vi "UHR-Fleezers Control (fpga) - 11.3h-c.vi"() -> ()   [LabVIEW 2012]
doc: "UHR-Fleezers Instrument Control Code (fpga)"
uses:
  <vilib>/Platform/TimedLoop/XDataNode/timing_clust.ctl
  <vilib>/Platform/TimedLoop/XDataNode/nitl_modes.ctl
  <vilib>/Platform/TimedLoop/XDataNode/wakeup.ctl
  <vilib>/rvi/eio/common/nirviEmuTemplateMethod_errors.vi
  <vilib>/rvi/interface/RandomDataEmulation/nirviRandomDataFPGAFIFO.vi
  <vilib>/rvi/interface/RandomDataEmulation/niFpgaRandomDataHandleErrors.vi
  <vilib>/rvi/Emulation/niFpgaSctlEmulationGetInTimedLoop.vi
  <vilib>/rvi/Emulation/niFpgaSctlEmulationGlobalWrite.vi
  <vilib>/rvi/Emulation/niFpgaSctlEmulationRegisterWithScheduler.vi
  <vilib>/rvi/Emulation/niFpgaSctlEmulationScheduler.vi
  <vilib>/Platform/TimedLoop/XDataNode/XDataNode.xnode
  <vilib>/eio/EIOMethodNode/EIOMethodNode.xnode
  <vilib>/eio/EIONode/EIONode.xnode
  <vilib>/rvi/DataTransferAndStorage/Container/XNode/niFpgaContainer.xnode
  <vilib>/rvi/interface/RandomDataEmulation/nirviRandomDataFpgaReadWriteTemplate.vi
  <vilib>/addons/control/pid/fpga.llb/XNode/niFpgaPID.xnode
  <vilib>/Platform/TimedLoop/XDataNode/XDNodeRunTimeDep.lvlib
panel:
  in  "Tab Control":T1(tab)=enum."Force FB"
  in  "Set 3":bool
  in  "Set 2":bool=TRUE
  in  "Set 1":bool=TRUE
  in  "Trap Pos to FIFO":bool
  in  "N of AI1 Int Acq Sets":i16=2 min=1 max=3 step=1
  out "AI Late Counter":u8
  in  "ai count":u16=400
  in  "+ phase":bool
  in  "Phase count adjustment":i16
  out "Relative phase":i16
  in  "AI to FIFO":bool
  out "BD1 Frequency Out 1":u64
  out "BD1 Frequency Out 2":u64
  out "Trap Pos FIFO Timeout":u16
  out "Trap AI FIFO Timeout":u16
  in  "Trap FIFO Set Timeout":i32
  in  "Tab Control 2":T2(tab)
  in  "RD":bool
  in  "FB1 output high":i16=3000
  in  "FB1 output low":i16
  in  "D1":i16
  in  "I1":i16=5
  in  "P1":i16=10
  in  "Swap F1 and F2":bool
  in  "Cont. Scan":bool
  in  "Abort scan":bool
  in  "Cycles per step":u64
  in  "Scan BD":bool
  in  "Number of scans":u16
  in  "Scan steps":u64
  in  "Scan freq.  increment":i64
  out "Scanning":bool
  in  "Start scan":bool
  in  "OSK Bd 1":bool
  in  "Reset Bd 1":bool
  in  "PMODE":bool
  in  "Direct RF Box \nCommunication":bool
  in  "Data BD 2":u8 format="%08b"
  in  "Data BD 1":u8 format="%08b"
  in  "Address":u8 format="%02x"
  in  "Update Data":bool
  in  "FPGA Controls\n RF Box":bool
  in  "Number Interlace Cycles":u8=2 min=1 max=3
  in  "Interlace Off Parameters":u8=1 min=1 max=3
  in  "Interlace ON/OFF":bool
  out "DIO Relative phase":i16
  in  "Phase count adjustment (DIO)":i16
  in  "+ phase (DIO)":bool
  out "DIO Late Counter":u8
  in  "DIO count 1 (ticks)":u16=400
  in  "DIO count 2 (ticks)":u16=400
  in  "DIO count 3 (ticks)":u16=400
  out "AI2 Y Sum Set 2":i16
  out "AI2 Y Sum Set 1":i16
  in  "FB Setpoint Set 1":i16 min=0 step=1
  in  "FB Reset Set 1":bool
  in  "FB On/Off Set 1":bool
  in  "FB Reset Set 2":bool
  in  "FB On/Off Set 2":bool
  in  "FB Setpoint Set 2":i16 min=0 step=1
  out "Scan I":u64
  in  "Amp switch delay":u16=5
  in  "BD 2 Amplitude 1":u16
  in  "BD 1 Amplitude 1":u16
  in  "BD 2 Frequency 1":u64
  in  "BD 1 Frequency 1":u64
  in  "BD 2 Amplitude 2":u16
  in  "BD 1 Amplitude 2":u16
  in  "BD 2 Frequency 2":u64
  in  "BD 1 Frequency 2":u64
  in  "BD 2 Amplitude 3":u16
  in  "BD 1 Amplitude 3":u16
  in  "BD 2 Frequency 3":u64
  in  "BD 1 Frequency 3":u64
  in  "FB2 output high":fxp<+/-,16,1>=0.999969482421875
  in  "FB2 output low":fxp<+/-,16,1>=-1.0
  in  "P2":fxp<+/-,16,8> format="%.11g"
  in  "I2":fxp<+/-,16,8>=10.0 format="%.11g"
  in  "D2":fxp<+/-,16,8> format="%.11g"
  in  "Negate Diff?":bool
  in  "Diff FB Measurement?":bool
  in  "FB Trig Integrate":u32=1
  out "TTrig?":bool
  in  "TTrig Negate Pos":bool=TRUE
  out "Trap Pos FB Int Signal":fxp<+/-,24,9> format="%.18g"
  out "Trap Pos FB Int-Norm Signal":fxp<+/-,16,1> format="%.16g"
  in  "FPGA TTrig Thresh":i64
  in  "FPGA Trap Trig":bool
  out "Trap Pos FB Action":i64
  in  "Trap Pos. FB Offset Factor":i64
  in  "Trap Pos. FB Mult Factor":i64=2
  in  "Trap Pos. FB Reset":bool
  in  "Trap Pos FB Monitor T1 or T2":bool
  in  "AI1 X Scale":u16
  in  "Trap Pos FB Int Count":u16=100
  in  "Trap Pos FB Negate Action":bool
  out "AI1 X Set 2":fxp<+/-,16,1>
  out "AI1 X Set 1":fxp<+/-,16,1>
  in  "Trap Pos. FB SP":fxp<+/-,16,1>
  in  "Force feedback":bool
  out "TTrig Sig":i64
  out "TTrig Fin Thresh":i64
  in  "1D or 2D Scan?":bool
  in  "Abort scan (MCL)":bool
  in  "MCL Scan Axis":bool
  in  "Cont. Scan (MCL)":bool
  out "Scan I (MCL)":u64
  in  "Number of scans (MCL)":u16
  out "Scanning MCL":bool
  in  "Scan steps (MCL)":u64
  in  "Cycles per step (MCL)":u64
  in  "Scan freq.  increment (MCL)":i16
  in  "Start scan (MCL)":bool
  in  "AO2":i16
  in  "AO1":i16
  out "MCL Late Counter":u8
  in  "MCL count":u32=800
  out "MCL Relative Phase":i16
  in  "Phase count adjustment (MCL)":i16
  in  "+ phase (MCL)":bool
  out "APD3 out state":bool
  in  "APD Gate Operating Mode":u8 max=2 step=1
  in  "Invert APD Gate":bool
  in  "APD Gate OFF Count":u16=100
  in  "APD Gate ON Count":u16=300
  out "APD 1 Gate Late Counter":u8
  out "APD 1 Gate Relative Phase":i16
  in  "Phase count adjustment (APD 1 Gate)":i16
  in  "+ phase (APD 1 Gate)":bool
  out "APD 2 Counts 0":u32
  out "APD 2 Counts 1":u32
  out "APD 1 Counts 0":u32
  out "APD 1 Counts 1":u32
  out "APD1 out state":bool
  in  "APD AO scale factor":i16=1
  in  "APD to FIFO":bool
  in  "APD Acq Rate Count":u32=20000000
  out "APD Acq Late Counter":u8
  out "APD Acq Relative Phase":i16
  in  "Phase Count Adjustment (APD Acq)":i16
  in  "+ phase (APD Acq)":bool
  in  "Phase count adjustment (APD 2 Gate)":i16
  out "APD 2 Gate Late Counter":u8
  out "APD 2 Gate Relative Phase":i16
  in  "+ phase (APD 2 Gate)":bool
  out "APD2 out state":bool
  out "APD 3 Counts 0":u32
  out "APD 3 Counts 1":u32
  out "APD 3 Gate Late Counter":u8
  in  "Phase count adjustment (APD 3 Gate)":i16
  out "APD 3 Gate Relative Phase":i16
  in  "+ phase (APD 3 Gate)":bool
  in  "D3":i16
  in  "I3":i16=5
  in  "P3":i16=10
  in  "Green Filter Flipper":bool
  in  "Green FB Count":u16=1200
  out "Green Late Counter":u8
  out "Green FB Relative Phase":i16
  in  "Phase count adjustment (Green FB)":i16=10
  in  "+ phase (Green FB)":bool
  out "Green FB Sum":i16
  in  "Green int current ON count adj":u16=150
  in  "Current Out":u16=30000
  in  "Green FB On/Off":bool
  in  "Green FB Setpoint":i16=250 min=0 step=1
  in  "Green FB Reset":bool
  in  "Operating Mode 2":u8=2 max=2 step=1
  in  "Invert GI 2":bool
  in  "Green interlace OFF count 2":u16=900
  in  "Green interlace ON count 2":u16=300
  out "GI Late Counter 2":u8
  out "GI Relative phase 2":i16
  in  "Phase count adjustment (GI) 2":i16=20
  in  "+ phase (GI) 2":bool
  in  "Green interlace OFF count":u16=100
  out "GI Relative phase":i16
  in  "Phase count adjustment (GI)":i16
  in  "+ phase (GI)":bool
  in  "Green interlace ON count":u16=300
  out "GI Late Counter":u8
  in  "Invert GI":bool
  in  "Operating Mode":u8 max=2 step=1
  in  "+ phase (RI)":bool
  out "RI Relative phase":i16
  out "RI Late Counter":u8
  in  "Red interlace ON count":u16=300
  in  "Red interlace OFF count":u16=100
  in  "Invert RI":bool
  in  "Red Laser Operating Mode":u8 max=2 step=1
  in  "Phase count adjustment (RI)":i16
  out "Red FB Intensity":i16
  in  "Phase count adjustment (Red FB)":i16=10
  in  "Red FB Count":u16=1200
  out "Red Late Counter":u8
  out "Red FB Relative Phase":i16
  in  "+ phase (Red FB)":bool
  in  "Phase count adjustment (RI) 2":i16=20
  in  "Red int current ON count adj":u16=150
  in  "RI Current Out":u16=30000
  in  "Red FB On/Off":bool
  in  "D4":i16
  in  "I4":i16=5
  in  "P4":i16=10
  in  "Red FB Setpoint":i16=250 min=0 step=1
  in  "Red FB Reset":bool
  in  "RI Operating Mode 2":u8=2 max=2 step=1
  in  "Invert RI 2":bool
  in  "Red interlace OFF count 2":u16=900
  in  "Red interlace ON count 2":u16=300
  out "RI Late Counter 2":u8
  out "RI Relative phase 2":i16
  in  "+ phase (RI) 2":bool
  in  "Phase count adjustment (BI AO)":i16=20
  in  "Blue current ON count adj (AO)":u16=150
  in  "BI Current Out":i16=30000
  in  "Blue FB On/Off":bool
  in  "D5":i16
  in  "I5":i16=5
  in  "P5":i16=10
  in  "Blue FB Setpoint":i16=250 min=0 step=1
  in  "Blue FB Reset":bool
  in  "BI Operating Mode (AO)":u8=2 max=2 step=1
  in  "Invert BI (AO)":bool
  in  "Blue OFF count (AO)":u16=900
  in  "Blue ON count (AO)":u16=300
  out "BI Late Counter (AO)":u8
  out "BI Relative phase (AO)":i16
  in  "+ phase (BI AO)":bool
  in  "Phase count adjustment (BI D)":i16
  in  "Blue Laser Operating Mode (D)":u8 max=2 step=1
  in  "Invert BI (D)":bool
  in  "Blue interlace OFF count (D)":u16=100
  in  "Blue interlace ON count (D)":u16=300
  out "Blue Late Counter (D)":u8
  out "BI Relative phase (D)":i16
  in  "+ phase (BI D)":bool
  out "Blue Intensity":i16
  in  "Phase count adjustment (Blue Int)":i16=10
  in  "Blue Int Count":u16=1200
  out "Blue Int Late Counter":u8
  out "Blue Int Relative Phase":i16
  in  "+ phase (Blue Int)":bool
  # "Only one of these can be on\nat a time:"
  # "Raster Scan AOD"
  # "1 (X)"
  # "2 (Y)"
  # "IR Intensity Feedback (RF BD 1)"
  # "FB Gains Set 1"
  # "FB output range 1"
  # "FB Triggering Excitation Laser"
  # "Trap Pos. FB Gains"
  # "Trap Pos. FB Range"
  # "AO1 (Y)"
  # "2D"
  # "1D"
  # "AO2 (X)"
  # "APD AO for aligning"
  # "Detection Loop"
  # "Green fluorescent laser digital gate interlacing loop"
  # "0 Forced ON\n1 Forced OFF\n2 Interlacing"
  # "Green FB Gains"
  # "Red fluorescent laser digital gate interlacing loop"
  # "Detection Loop"
  # "0 Forced ON\n1 Forced OFF\n2 Interlacing"
  # "Analog/FB Control Loop\n(Disabled)"
  # "Digital Control Loop"
  # "Blue laser intensity reading"
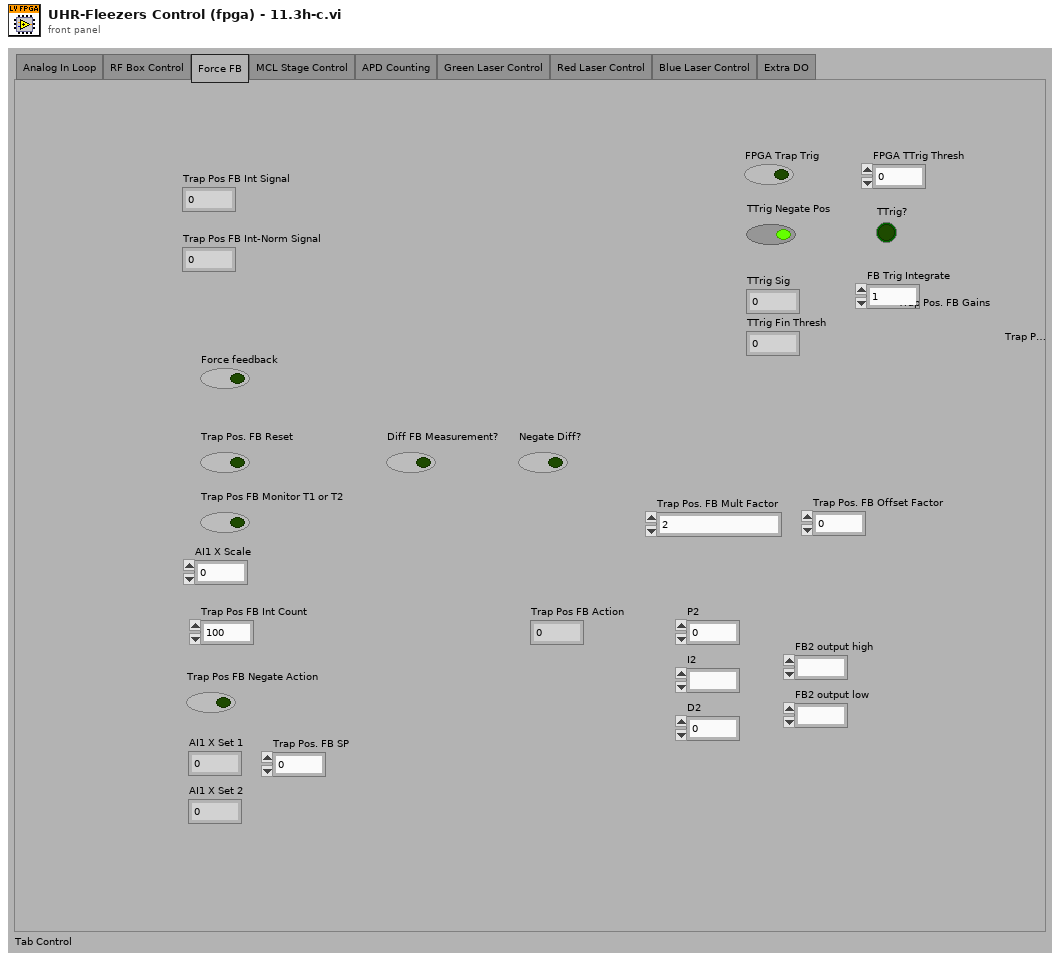
[diagram p1: front panel]
types:
  T1 = enum32{"Analog In Loop", "RF Box Control", "Force FB", "MCL Stage Control", "APD Counting", "Green Laser Control", "Red Laser Control", "Blue Laser Control", "Extra DO"}
  T2 = enum32{"Controls", "Interlacing Frequency and Amplitude Values"}
  T3 = typedef "XDNodeRunTimeDep.lvlib/timing_clust.ctl" = cluster{"Expected End [f-1]":u64, "Actual End [f-1]":u64, "Finished Late? [f-1]":bool, "Expected End [i-1]":u64, "Actual End [i-1]":u64, "Finished Late? [i-1]":bool, "Expected Start [i]":u64, "Actual Start [i]":u64, "Expected Start [f]":u64, "Actual Start [f]":u64, "Source Name":string, "Structure Name":string, "Period":i64, "Deadline":i64, "Offset":i64, "Start":i64, "Priority":i32, "Timeout":i32, "Mode":T4, "Wakeup Reason":T5, "Error":errorcluster, "Source Type":string, "Secondary Source Type":string, "Global End Time":u64, "Global Start Time":u64, "Frame Duration":u64, "Iteration Duration":u64, "Assigned CPU":i32, "I/O Scan Engine Mode":u32}
  T4 = typedef "XDNodeRunTimeDep.lvlib/nitl_modes.ctl" = enum32{"No Change", "Process missed periods, maintain original phase", "Discard missed periods, maintain original phase", "Process missed periods, ignore original phase", "Discard missed periods, ignore original phase"}
  T5 = typedef "XDNodeRunTimeDep.lvlib/wakeup.ctl" = enum32{"Normal", "Aborted", "Asynchronous wakeup", "Timing source error", "Timed loop error", "Timeout"}
  T6 = cluster{"proportional gain (Kc)":i16, "integral gain (Kc*Ts/Ti)":i16, "derivative gain (Kc*Td/Ts)":i16}
  T7 = cluster{"FB1 output high":i16, "FB1 output low":i16}
  T8 = cluster{"P2":fxp<+/-,16,8>, "I2":fxp<+/-,16,8>, "D2":fxp<+/-,16,8>}
  T9 = cluster{"FB2 output high":fxp<+/-,16,1>, "FB2 output low":fxp<+/-,16,1>}
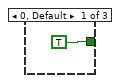
[diagram p3: hidden frame]
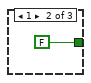
[diagram p4: hidden frame]
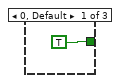
[diagram p5: hidden frame]
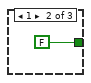
[diagram p6: hidden frame]
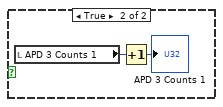
[diagram p7: hidden frame]
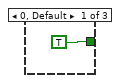
[diagram p8: hidden frame]
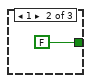
[diagram p9: hidden frame]
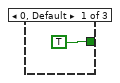
[diagram p11: hidden frame]
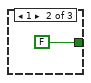
[diagram p12: hidden frame]
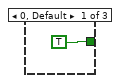
[diagram p13: hidden frame]
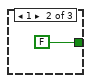
[diagram p14: hidden frame]
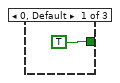
[diagram p15: hidden frame]
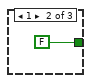
[diagram p16: hidden frame]
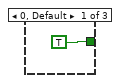
[diagram p18: hidden frame]
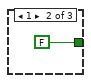
[diagram p19: hidden frame]
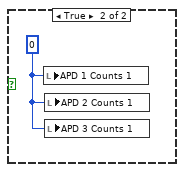
[diagram p20: hidden frame]
diagram:
  w3 = FALSE
  # "timing array current index"
  # "timing array"
  # "timing counter (phase adjusted here)"
  # "late counter"
  n1 = flat-sequence "FPGA initialization to do before running any of the loops" {
    tunnel: [u16 0 ("DIO count 3 (ticks)")] -> w2
    tunnel: [w12] -> _
    frame #0 {
      # "Start up expansion chassis early\nto avoid delays later"
      # "This pin controls udclk on the RF boards.\nWhen initially configuring the boards, this pin needs to be\nconfigured as a high impedance input.  Later it will be switched\nto an output."
      # "Initial setting of DIO data and \naddress to low (before reset).  \nThis needs to happen before the other\ncontrol method loops execute."
      n2 = xnode "FPGA I/O Node"("Chassis2/Mod4/AO0"=u16 0) -> ("Chassis2/Mod1/AI0"=w12:i16)  [unwired: 2 in, 2 out]
      n3 = xnode "FPGA I/O Method Node"("Enable"=FALSE) -> ()  [unwired: 1 in, 1 out]
      n4 = xnode "FPGA I/O Node"("Connector1/DIO0"=FALSE, "Connector1/DIO1"=FALSE, "Connector1/DIO2"=FALSE, "Connector1/DIO3"=FALSE, "Connector1/DIO4"=FALSE, "Connector1/DIO5"=FALSE, "Connector1/DIO6"=FALSE, "Connector1/DIO7"=FALSE, "Connector1/DIO8"=FALSE, "Connector1/DIO9"=FALSE, "Connector1/DIO10"=FALSE, "Connector1/DIO11"=FALSE, "Connector1/DIO12"=FALSE, "Connector1/DIO13"=FALSE, "Connector1/DIO15"=FALSE, "Connector1/DIO20"=FALSE, "Connector1/DIO21"=FALSE, "Connector1/DIO22"=FALSE, "Connector1/DIO23"=FALSE, "Connector1/DIO24"=FALSE, "Connector1/DIO25"=FALSE, "Connector1/DIO26"=FALSE, "Connector1/DIO27"=FALSE, "Connector1/DIO14"=FALSE) -> ()  [unwired: 24 in, 24 out]
    }
  }
  n5 = local read "AO1"() -> (w9:i16)
  n6 = local read "AO2"() -> (w8:i16)
  n7 = node-c288() -> (w7:T3)  [unwired: 1 in]
  n8 = timed-loop "RF box board DIO control: control bits" {
    timing: w7 -> [_]
    timing-out: [_] -> w6
    tunnel: [w42] -> _
    tunnel: w2 -> [w42]
    stop <- FALSE stop-if-true
    n9 = xnode "FPGA I/O Node"("Connector1/DIO16"="RD", "Connector1/DIO17"="PMODE", "Connector1/DIO18"="OSK Bd 1", "Connector1/DIO19"="Reset Bd 1", "Connector0/DIO3"="Green Filter Flipper") -> ()  [unwired: 5 in, 5 out]
  }
  n10 = while "RF box board DIO control: parallel communication" {
    shift-right: [w55] -> _
    shift-left: w2 -> [w54]
    shift-right: [w53] -> _
    shift-left: FALSE ("Swap F1 and F2") -> [w52]
    stop <- FALSE stop-if-true
    n11 = flat-sequence {
      tunnel: w52 -> [w59]
      tunnel: w54 -> [w57]
      tunnel: [w59] -> w51
      tunnel: [w58] -> w50
      tunnel: [w57] -> w49
      tunnel: [w65] -> w55
      tunnel: [w64] -> w53
      tunnel: w51 -> [w63]
      tunnel: w50 -> [w61]
      tunnel: w49 -> [w60]
      frame #0 {
        n12 = call "Loop Timer"("Count(Ticks)"=w57) -> ("Tick Count(Ticks)"=w58:u16)
      }
      frame #1 {
        n13 = flat-sequence {
          tunnel: ["FPGA Controls\n RF Box"] -> w62
          tunnel: w63 -> [w66]
          tunnel: [w106] -> w65
          tunnel: [w119] -> w64
          tunnel: w62 -> [w118]
          tunnel: w61 -> [w112]
          tunnel: w60 -> [w109]
          frame #0 {
            n14 = case shown="True" "FPGA Controls\n RF Box" {
              tunnel: w66 -> [_ w68]
              frame False {
              }
              frame True {
                n15 = flat-sequence {
                  tunnel: w68 -> [w74]
                  frame #0 {
                    n16 = First Call?() -> (First Call?: T/F=w69:bool)
                    n17 = case shown="True" w69 {
                      frame False {
                      }
                      frame True {
                        # "If first time data updated, be sure to set WR high and UDCLK low\nbefore setting data and address bits."
                        n18 = xnode "FPGA I/O Method Node"("Enable"=TRUE) -> ("FPGA I/O Out"=w71:refnum<k21>)  [unwired: 1 in]
                        n19 = xnode "FPGA I/O Node"("Connector1/DIO15"=TRUE) -> ()  [unwired: 1 in, 1 out]
                        n20 = xnode "FPGA I/O Node"("I/O Item"=FALSE ("Connector1/DIO30"), "FPGA I/O In"=w71) -> ()  [unwired: 1 out]
                      }
                    }
                  }
                  frame #1 {
                    n21 = flat-sequence {
                      tunnel: w74 -> [w75]
                      frame #0 {
                        # "switch frequency"
                        n22 = xnode "FPGA I/O Node"("Connector1/DIO36"=w75) -> ()  [unwired: 1 in, 1 out]
                      }
                      frame #1 {
                        n23 = call "Wait4"("Count(Ticks)"="Amp switch delay") -> ()  [unwired: 1 out]
                      }
                      frame #2 {
                        # "switch amplitude"
                        # "send udclk high"
                        n24 = xnode "FPGA I/O Node"("Connector1/DIO30"=TRUE ("Connector1/DIO15")) -> ()  [unwired: 1 in, 1 out]
                      }
                      frame #3 {
                        # "send udclk low"
                        n25 = xnode "FPGA I/O Node"("Connector1/DIO30"=FALSE ("Connector1/DIO15")) -> ()  [unwired: 1 in, 1 out]
                      }
                    }
                  }
                }
              }
            }
          }
          frame #1 {
            # "This is the prior cycle's on time"
            # "increment timing\nindex, reset to 0 if \nend of matrix"
            # "Reset to begginning (1) when number of cycles reached."
            # "timing index"
            # "build byte stacks for writing data\n(must correspond to addresses array constant)"
            # "Timing housekeeping"
            # "Adjust phase if late\n(maintains constant phase relationship between cycles)"
            n26 = Bundle("FB1 output high"="FB1 output high", "FB1 output low"="FB1 output low") -> (w79:T7)  [unwired: 1 in]
            n27 = Bundle("P1"="P1", "I1"="I1", "D1"="D1") -> (w80:cluster{"P1":i16, "I1":i16, "D1":i16})  [unwired: 1 in]
            n28 = feedback #1(u8 0 ("t")) -> (w115:u8)
            n29 = Increment(x=w115) -> (x+1=w159:u8)
            n30 = Increment(x="Number Interlace Cycles") -> (x+1=w154:u8)
            n31 = Equal?(x=w159, y=w154) -> (x = y?=w161:bool)
            n32 = Select(t=u8 1, s=w161, f=w159) -> (s? t:f=w114:u8)
            n33 = feedback-in #1(w114) -> ()
            n34 = Increment(x=w114) -> (x+1=w156:u8)
            n35 = Equal?(x=w156, y=w154) -> (x = y?=w157:bool)
            n36 = Select(t=u8 1, s=w157, f=w156) -> (s? t:f=w153:u8)
            n37 = Select(t=w153, s="Interlace ON/OFF", f="Interlace Off Parameters") -> (s? t:f=w137:u8)
            n38 = case shown="1, Default" w137 {
              tunnel: [w233 "BD 1 Frequency 2" "BD 1 Frequency 3"] -> w149
              tunnel: [w232 "BD 2 Frequency 2" "BD 2 Frequency 3"] -> w138
              tunnel: ["BD 2 Amplitude 1" "BD 2 Amplitude 2" "BD 2 Amplitude 3"] -> w94
              tunnel: [w221 w392 "BD 1 Amplitude 3"] -> w97
              tunnel: w80 -> [w195 w389 _]
              tunnel: w79 -> [w196 w388 _]
              frame 1, Default {
                w212 = fxp<+/-,24,9> 0.0 ("AI1 X Set 2")
                w205 = u16 0
                w228 = u64 0 ("f")
                # "This signal integration happens no matter what\nso that correct setpoints can be chosen before \nturning on the FB."
                # "Trap 1"
                n39 = local read "AI1 X Set 2"() -> (w208:fxp<+/-,16,1>)
                n40 = local read "AI1 X Set 1"() -> (w209:fxp<+/-,16,1>)
                n41 = local read "Scanning"() -> (w234:bool)
                n42 = Or(x=w234, y="Start scan") -> (x .or. y?=w226:bool)
                n43 = case shown="False" "Diff FB Measurement?" {
                  tunnel: w208 -> [w242 w251]
                  tunnel: w209 -> [w241 w252]
                  tunnel: [w239 w243] -> w210
                  frame False {
                    n44 = Select(t=w241, s="Trap Pos FB Monitor T1 or T2", f=w242) -> (s? t:f=w239:fxp<+/-,16,1>)
                  }
                  frame True {
                    n45 = Subtract(x=w252, y=w251) -> (x-y=w244:fxp<+/-,17,2>)
                    n46 = Not(x="Negate Diff?") -> (.not. x?=w250:bool)
                    n47 = Boolean To (0,1)(Boolean="Negate Diff?") -> (0, 1=w248:i16)
                    n48 = Boolean To (0,1)(Boolean=w250) -> (0, 1=w249:i16)
                    n49 = Negate(x=w248) -> (-x=w247:i16)
                    n50 = Add(x=w247, y=w249) -> (x+y=w245:i16)
                    n51 = Multiply(x=w245, y=w244) -> (x*y=w243:fxp<+/-,32,17>)
                  }
                }
                n52 = Not(x="Abort scan") -> (.not. x?=w224:bool)
                n53 = And(x=w224, y=w226) -> (x .and. y?=w223:bool)
                n54 = case "For raster scanning" shown="True" w223 {
                  tunnel: [u64 0 w378] -> w229
                  tunnel: "Start scan" -> [_ w363]
                  frame False {
                    n55 = local write "Scanning"(FALSE ("scanning")) -> ()
                  }
                  frame True {
                    w347 = i64 0
                    w346 = u64 0
                    # "scan incr."
                    # "freq. incr. mult."
                    # "count steps"
                    # "count number of cycles"
                    n56 = feedback #2(w346) -> (w375:u64)
                    n57 = Select(t=w346, s=w363, f=w375) -> (s? t:f=w377:u64)
                    n58 = Increment(x=w377) -> (x+1=w374:u64)
                    n59 = Greater?(x="Cycles per step", y=w374) -> (0:w356:bool)
                    n60 = Select(t=w374, s=w356, f=w346) -> (s? t:f=w373:u64)
                    n61 = feedback-in #2(w373) -> ()
                    n62 = feedback #3(w346) -> (w372:u64)
                    n63 = Select(t=w346, s=w363, f=w372) -> (s? t:f=w367:u64)
                    n64 = Increment(x=w367) -> (x+1=w371:u64)
                    n65 = Add(x="Scan steps", y="Scan steps") -> (x+y=w370:u64)
                    n66 = Select(t=w367, s=w356, f=w371) -> (s? t:f=w351:u64)
                    n67 = Greater?(x=w370, y=w351) -> (0:w350:bool)
                    n68 = Select(t=w351, s=w350, f=w346) -> (s? t:f=w368:u64)
                    n69 = feedback-in #3(w368) -> ()
                    n70 = Equal?(x="Scan steps", y=w351) -> (x = y?=w355:bool)
                    n71 = Greater?(x="Scan steps", y=w367) -> (0:w366:bool)
                    n72 = feedback #4(w347) -> (w369:i64)
                    n73 = Select(t=w347, s=w363, f=w369) -> (s? t:f=w353:i64)
                    n74 = Increment(x=w353) -> (x+1=w365:i64)
                    n75 = Decrement(x=w353) -> (x-1=w364:i64)
                    n76 = Select(t=w365, s=w366, f=w364) -> (s? t:f=w354:i64)
                    n77 = Select(t=w353, s=w355, f=w354) -> (s? t:f=w352:i64)
                    n78 = Select(t=w353, s=w356, f=w352) -> (s? t:f=w348:i64)
                    n79 = Select(t=w348, s=w350, f=w347) -> (s? t:f=w349:i64)
                    n80 = feedback-in #4(w349) -> ()
                    n81 = feedback #5(w346) -> (w362:u64)
                    n82 = Select(t=w346, s=w363, f=w362) -> (s? t:f=w358:u64)
                    n83 = Increment(x=w358) -> (x+1=w359:u64)
                    n84 = Select(t=w358, s=w350, f=w359) -> (s? t:f=w357:u64)
                    n85 = Greater?(x="Number of scans", y=w357) -> (0:w343:bool)
                    n86 = Multiply(x="Scan freq.  increment", y=w353) -> (x*y=w378:i64)
                    n87 = Select(t=TRUE, s="Cont. Scan", f=w343) -> (s? t:f=w342:bool)
                    "Scanning" <- w342
                    n88 = Select(t=w357, s=w342, f=w346) -> (s? t:f=w360:u64)
                    n89 = feedback-in #5(w360) -> ()
                    n90 = Increment(x=w357) -> (x+1=→"Scan I":u64)
                  }
                }
                n91 = feedback #6(w205) -> (w204:u16)
                n92 = Increment(x=w204) -> (x+1=w206:u16)
                n93 = Greater Or Equal?(x=w206, y="Trap Pos FB Int Count") -> (x >= y?=w197:bool)
                n94 = Select(t=w205, s=w197, f=w206) -> (s? t:f=w207:u16)
                n95 = feedback-in #6(w207) -> ()
                n96 = feedback #7(w212) -> (w211:fxp<+/-,24,9>)
                n97 = Add(x=w210, y=w211) -> (x+y=w203:fxp<+/-,24,9>)
                n98 = case "For intensity feedback" shown="True" "FB On/Off Set 1" {
                  tunnel: "BD 1 Amplitude 1" -> [w380 _]
                  tunnel: [w380 w384] -> w221
                  tunnel: w196 -> [_ w381]
                  tunnel: w195 -> [_ w382]
                  frame False {
                  }
                  frame True {
                    n99 = local read "AI2 Y Sum Set 1"() -> (w385:i16)
                    n100 = call "Slower PID.vi"("process variable"=w385, "reset?"="FB Reset Set 1", "setpoint"="FB Setpoint Set 1", "PID gains (x 2^8)"=w382, "output range"=w381) -> ("output"=w386:i16)  [unwired: 10 out]
                    n101 = To Unsigned Word Integer(number=w386) -> (unsigned 16bit integer=w384:u16)
                  }
                }
                n102 = Select(t=w212, s=w197, f=w203) -> (s? t:f=w215:fxp<+/-,24,9>)
                n103 = feedback-in #7(w215) -> ()
                n104 = Divide(x=w203, y="Trap Pos FB Int Count") -> (x/y=w198:fxp<+/-,16,1>)
                n105 = feedback #8(fxp<+/-,24,9> 0.0 ("AI1 X Set 2")) -> (w216:fxp<+/-,24,9>)
                n106 = Select(t=w203, s=w197, f=w216) -> (s? t:f=w217:fxp<+/-,24,9>)
                "Trap Pos FB Int Signal" <- w217
                n107 = feedback-in #8(w217) -> ()
                n108 = feedback #9(fxp<+/-,16,1> 0.0 ("Trap Pos FB Int-Norm Signal")) -> (w200:fxp<+/-,16,1>)
                n109 = Select(t=w198, s=w197, f=w200) -> (s? t:f=w199:fxp<+/-,16,1>)
                "Trap Pos FB Int-Norm Signal" <- w199
                n110 = feedback-in #9(w199) -> ()
                n111 = case "For position feedback" shown="True" "Force feedback" {
                  tunnel: [i64 0 w258] -> w218
                  tunnel: w198 -> [_ w255]
                  tunnel: w197 -> [_ w254]
                  frame False {
                  }
                  frame True {
                    n112 = feedback #10(i64 0) -> (w257:i64)
                    n113 = case shown="True" w254 {
                      tunnel: [w259 w273] -> w258
                      tunnel: w257 -> [w259 _]
                      tunnel: w255 -> [_ w267]
                      frame False {
                      }
                      frame True {
                        w277 = u32 0
                        n114 = Bundle("P2"="P2", "I2"="I2", "D2"="D2") -> (w263:T8)  [unwired: 1 in]
                        n115 = Bundle("FB2 output high"="FB2 output high", "FB2 output low"="FB2 output low") -> (w260:T9)  [unwired: 1 in]
                        n116 = xnode ("PID")("process variable"=w267, "reset?"="Trap Pos. FB Reset", "setpoint"="Trap Pos. FB SP", "PID gains"=w263, "output range"=w260) -> ("output"=w289:fxp<+/-,16,1>)
                        n117 = Negate(x=w289) -> (-x=w288:fxp<+/-,17,2>)
                        n118 = Select(t=w288, s="Trap Pos FB Negate Action", f=w289) -> (s? t:f=w285:fxp<+/-,17,2>)
                        n119 = Scale By Power Of 2(n=u32 15, x=u32 1) -> (x*2^n=w282:u32)
                        n120 = Multiply(x=w285, y=w282) -> (x*y=w281:fxp<+/-,17,17>)
                        n121 = To Quad Integer(1:w281) -> (0:w293:i64)
                        "Trap Pos FB Action" <- w293
                        n122 = Multiply(x=w293, y="Trap Pos. FB Mult Factor") -> (x*y=w291:i64)
                        n123 = Add(x=w291, y="Trap Pos. FB Offset Factor") -> (x+y=w273:i64)
                        n124 = feedback #11() -> (w274:i64)  [unwired: 1 in]
                        n125 = Add(x=w273, y=w274) -> (x+y=w271:i64)
                        n126 = feedback #12(w277) -> (w279:u32)
                        n127 = Increment(x=w279) -> (x+1=w268:u32)
                        n128 = Greater Or Equal?(x=w268, y="FB Trig Integrate") -> (x >= y?=w269:bool)
                        n129 = Select(t=i64 0, s=w269, f=w271) -> (s? t:f=w275:i64)
                        n130 = feedback-in #11(w275) -> ()
                        n131 = Select(t=w277, s=w269, f=w268) -> (s? t:f=w278:u32)
                        n132 = feedback-in #12(w278) -> ()
                        n133 = And(x=w269, y="FPGA Trap Trig") -> (x .and. y?=w276:bool)
                        n134 = case "Trap FB trigger excitation laser ON" shown="True" w276 {
                          tunnel: w271 -> [_ w297]
                          tunnel: w268 -> [_ w295]
                          frame False {
                          }
                          frame True {
                            n135 = Not(x="TTrig Negate Pos") -> (.not. x?=w304:bool)
                            n136 = Boolean To (0,1)(Boolean="TTrig Negate Pos") -> (0, 1=w302:i16)
                            n137 = Boolean To (0,1)(Boolean=w304) -> (0, 1=w303:i16)
                            n138 = Negate(x=w302) -> (-x=w301:i16)
                            n139 = Add(x=w301, y=w303) -> (x+y=w300:i16)
                            n140 = Multiply(x=w300, y=w297) -> (x*y=w299:i64)
                            "TTrig Sig" <- w299
                            n141 = Multiply(x="FPGA TTrig Thresh", y=w295) -> (x*y=w296:i64)
                            "TTrig Fin Thresh" <- w296
                            n142 = Greater Or Equal?(x=w299, y=w296) -> (x >= y?=w298:bool)
                            n143 = case shown="True" w298 {
                              frame False {
                              }
                              frame True {
                                w307 = TRUE ("Green FB On/Off")
                                w309 = u8 2 ("Operating Mode")
                                n144 = local write "Operating Mode 2"(w309) -> ()
                                n145 = local write "Operating Mode"(w309) -> ()
                                n146 = local write "Green FB On/Off"(w307) -> ()
                                n147 = local write "FPGA Trap Trig"(FALSE ("FPGA Trap Trig")) -> ()
                                "TTrig?" <- w307
                              }
                            }
                          }
                        }
                      }
                    }
                    n148 = feedback-in #10(w258) -> ()
                  }
                }
                n149 = Select(t=w228, s="Scan BD", f=w229) -> (s? t:f=w227:u64)
                n150 = Select(t=w229, s="Scan BD", f=w228) -> (s? t:f=w230:u64)
                n151 = Add(x=w227, y="BD 2 Frequency 1") -> (x+y=w232:u64)
                n152 = Compound Arithmetic op=ADD("BD 1 Frequency 1", w218, w230) -> (w233:u64)
                "BD1 Frequency Out 1" <- w233
              }
              frame 2 {
                # "Trap 2"
                n153 = case shown="True" "FB On/Off Set 2" {
                  tunnel: [w396 w399] -> w392
                  tunnel: "BD 1 Amplitude 2" -> [w396 _]
                  tunnel: w389 -> [_ w398]
                  tunnel: w388 -> [_ w397]
                  frame False {
                  }
                  frame True {
                    n154 = local read "AI2 Y Sum Set 2"() -> (w402:i16)
                    n155 = call "Slower PID.vi"("process variable"=w402, "reset?"="FB Reset Set 2", "setpoint"="FB Setpoint Set 2", "PID gains (x 2^8)"=w398, "output range"=w397) -> ("output"=w400:i16)  [unwired: 10 out]
                    n156 = To Unsigned Word Integer(number=w400) -> (unsigned 16bit integer=w399:u16)
                  }
                }
                "BD1 Frequency Out 2" <- "BD 1 Frequency 2"
              }
              frame 3 {
                # "Fluorescence period"
              }
            }
            n157 = feedback-in #13(w112) -> ()
            n158 = feedback #13(w112) -> (w111:u16)
            n159 = Select(t=w114, s="Interlace ON/OFF", f="Interlace Off Parameters") -> (s? t:f=w152:u8)
            n160 = Subtract(x=w112, y=w111) -> (x-y=w110:u16)
            n161 = Subtract "The error"(x=w110, y=w109) -> (x-y=w87:u16)
            n162 = case shown="1, Default" w152 {
              tunnel: ["DIO count 1 (ticks)" "DIO count 2 (ticks)" "DIO count 3 (ticks)"] -> w108
              frame 1, Default {
              }
              frame 2 {
              }
              frame 3 {
              }
            }
            n163 = Number To Boolean Array(number=w87) -> (Boolean array=w88:bool[])
            n164 = Or Array Elements(Boolean array=w88) -> (logical OR=w86:bool)
            n165 = Boolean To (0,1)(Boolean=w86) -> (0, 1=w93:i16)
            n166 = To Unsigned Byte Integer(number=w93) -> (unsigned 8bit integer=w90:u8)
            n167 = feedback #14(u8 0) -> (w91:u8)
            n168 = Add(x=w90, y=w91) -> (x+y=w89:u8)
            "DIO Late Counter" <- w89
            n169 = feedback-in #14(w89) -> ()
            n170 = Subtract(x=w108, y=w87) -> (x-y=w107:u16)
            n171 = Split Number(x=w149) -> (hi(x)=w148:u32, lo(x)=w147:u32)
            n172 = Split Number(x=w138) -> (hi(x)=w143:u32, lo(x)=w142:u32)
            n173 = Boolean To (0,1)(Boolean="+ phase (DIO)") -> (0, 1=w104:i16)
            n174 = Split Number(x=w148) -> (lo(x)=w146:u16)  [unwired: 1 out]
            n175 = Split Number(x=w147) -> (hi(x)=w145:u16, lo(x)=w144:u16)
            n176 = Split Number(x=w143) -> (lo(x)=w141:u16)  [unwired: 1 out]
            n177 = Split Number(x=w142) -> (hi(x)=w140:u16, lo(x)=w139:u16)
            n178 = Split Number(x=w97) -> (hi(x)=w99:u8, lo(x)=w98:u8)
            n179 = Split Number(x=w94) -> (hi(x)=w96:u8, lo(x)=w95:u8)
            n180 = Split Number(x=w146) -> (hi(x)=w136:u8, lo(x)=w135:u8)
            n181 = Split Number(x=w145) -> (hi(x)=w134:u8, lo(x)=w133:u8)
            n182 = Split Number(x=w141) -> (hi(x)=w129:u8, lo(x)=w128:u8)
            n183 = Split Number(x=w144) -> (hi(x)=w132:u8, lo(x)=w131:u8)
            n184 = Split Number(x=w140) -> (hi(x)=w127:u8, lo(x)=w126:u8)
            n185 = Split Number(x=w139) -> (hi(x)=w125:u8, lo(x)=w124:u8)
            n186 = Multiply(x=w104, y="Phase count adjustment (DIO)") -> (x*y=w100:i16)
            n187 = feedback #15(i16 0) -> (w102:i16)
            n188 = Subtract(x=w102, y=w100) -> (x-y=w101:i16)
            "DIO Relative phase" <- w101
            n189 = feedback-in #15(w101) -> ()
            n190 = Add(x=w107, y=w100) -> (x+y=w106:u16)
            n191 = Build Array "BD 1 A Stack"(w99, w98) -> (w121:u8[])
            n192 = Build Array "BD 2 A Stack"(w96, w95) -> (w120:u8[])
            n193 = Build Array "BD 1 nu Stack"(w136, w135, w134, w133, w132, w131) -> (w130:u8[])
            n194 = Build Array "BD 2 nu Stack"(w129, w128, w127, w126, w125, w124) -> (w123:u8[])
            n195 = case shown="2" w137 {
              tunnel: [w187 w190] -> w119
              tunnel: [u8 10 u8 4] -> w122
              tunnel: "Swap F1 and F2" -> [w188 w190]
              frame 2 {
                # "F2"
                n196 = Not(x=w188) -> (.not. x?=w187:bool)
              }
              frame 1, Default {
                # "low chooses F1"
                # "F1"
              }
            }
            n197 = case "If FPGA is controlling (toggling) RF synth" shown="True" w118 {
              tunnel: w130 -> [_ w166]
              tunnel: w123 -> [_ w165]
              tunnel: w122 -> [_ w164]
              tunnel: w121 -> [_ w163]
              tunnel: w120 -> [_ w162]
              frame False {
              }
              frame True {
                # "Write next amp.\n(wait until beginning of next loop iteration to update)"
                n198 = flat-sequence "Update the next F1 and F2 frequency value (the actual frequency won't change until FSK is switched).\nThen load the next amplitude value into buffer, but don't update it until the next cycle." {
                  tunnel: w166 -> [w169]
                  tunnel: w165 -> [w168]
                  tunnel: w164 -> [w167]
                  tunnel: w163 -> [w180]
                  tunnel: w162 -> [w179]
                  frame #0 {
                    n199 = for {
                      tunnel: w169 -> [w175] mode=indexing
                      tunnel: w168 -> [w174] mode=indexing
                      tunnel: w167 -> [w172]
                      i -> [w173]
                      # "Write next freq."
                      n200 = To Unsigned Byte Integer(number=w173) -> (unsigned 8bit integer=w170:u8)
                      n201 = Add(x=w172, y=w170) -> (x+y=w171:u8)
                      n202 = call "write to RF synth bd.vi"("Address Byte"=w171, "BD 2 Byte"=w174, "BD 1 Byte"=w175) -> ()
                    }
                  }
                  frame #1 {
                    # "send udclk high"
                    n203 = xnode "FPGA I/O Node"("Connector1/DIO30"=TRUE ("Connector1/DIO15")) -> ()  [unwired: 1 in, 1 out]
                  }
                  frame #2 {
                    n204 = xnode "FPGA I/O Node"("Connector1/DIO30"=FALSE ("Connector1/DIO15")) -> ()  [unwired: 1 in, 1 out]
                  }
                  frame #3 {
                    n205 = for {
                      tunnel: w180 -> [w186] mode=indexing
                      tunnel: w179 -> [w185] mode=indexing
                      tunnel: u8 33 -> [w183]
                      i -> [w184]
                      n206 = To Unsigned Byte Integer(number=w184) -> (unsigned 8bit integer=w181:u8)
                      n207 = Add(x=w183, y=w181) -> (x+y=w182:u8)
                      n208 = call "write to RF synth bd.vi"("Address Byte"=w182, "BD 2 Byte"=w185, "BD 1 Byte"=w186) -> ()
                    }
                  }
                }
              }
            }
          }
        }
      }
    }
  }
  n209 = while "RF box board direct communication loop" {
    tunnel: w2 -> [_]
    stop <- FALSE stop-if-true
    n210 = case "Whether to use direct communication method (only use one method at a time)" shown="True" "Direct RF Box \nCommunication" {
      frame False {
      }
      frame True {
        n211 = case shown="True" "Update Data" {
          frame False {
          }
          frame True {
            n212 = flat-sequence {
              frame #0 {
                n213 = First Call?() -> (First Call?: T/F=w411:bool)
                n214 = case shown="True" w411 {
                  frame False {
                  }
                  frame True {
                    # "If first time data updated, be sure to set WR high\nbefore setting data and address bits."
                    n215 = flat-sequence {
                      frame #0 {
                        n216 = xnode "FPGA I/O Node"("Connector1/DIO15"=TRUE) -> ()  [unwired: 1 in, 1 out]
                      }
                      frame #1 {
                        n217 = call "Wait"("Count(Ticks)"=u8 40 ("DO Delay 3 (Ticks)")) -> ()  [unwired: 1 out]
                      }
                    }
                  }
                }
              }
              frame #1 {
                n218 = Number To Boolean Array(number="Address") -> (Boolean array=w460:bool[])
                n219 = Number To Boolean Array(number="Data BD 1") -> (Boolean array=w461:bool[])
                n220 = Number To Boolean Array(number="Data BD 2") -> (Boolean array=w430:bool[])
                n221 = Index Array(array=w461, index=7) -> (element=w445:bool)
                n222 = Index Array(array=w461, index=6) -> (element=w444:bool)
                n223 = Index Array(array=w461, index=5) -> (element=w443:bool)
                n224 = Index Array(array=w461, index=4) -> (element=w442:bool)
                n225 = Index Array(array=w461, index=3) -> (element=w441:bool)
                n226 = Index Array(array=w461, index=2) -> (element=w440:bool)
                n227 = Index Array(array=w461, index=1) -> (element=w439:bool)
                n228 = Index Array(array=w461, index=0) -> (element=w438:bool)
                n229 = Index Array(array=w460, index=5) -> (element=w437:bool)
                n230 = Index Array(array=w460, index=4) -> (element=w436:bool)
                n231 = Index Array(array=w460, index=3) -> (element=w435:bool)
                n232 = Index Array(array=w460, index=2) -> (element=w434:bool)
                n233 = Index Array(array=w460, index=1) -> (element=w433:bool)
                n234 = Index Array(array=w460, index=0) -> (element=w432:bool)
                n235 = Index Array(array=w430, index=7) -> (element=w421:bool)
                n236 = Index Array(array=w430, index=6) -> (element=w420:bool)
                n237 = Index Array(array=w430, index=5) -> (element=w419:bool)
                n238 = Index Array(array=w430, index=4) -> (element=w418:bool)
                n239 = Index Array(array=w430, index=3) -> (element=w417:bool)
                n240 = Index Array(array=w430, index=2) -> (element=w416:bool)
                n241 = Index Array(array=w430, index=1) -> (element=w415:bool)
                n242 = Index Array(array=w430, index=0) -> (element=w414:bool)
                n243 = xnode "FPGA I/O Node"("Connector1/DIO0"=w445, "Connector1/DIO1"=w444, "Connector1/DIO2"=w443, "Connector1/DIO3"=w442, "Connector1/DIO4"=w441, "Connector1/DIO5"=w440, "Connector1/DIO6"=w439, "Connector1/DIO7"=w438, "Connector1/DIO8"=w437, "Connector1/DIO9"=w436, "Connector1/DIO10"=w435, "Connector1/DIO11"=w434, "Connector1/DIO12"=w433, "Connector1/DIO13"=w432, "Connector1/DIO20"=w421, "Connector1/DIO21"=w420, "Connector1/DIO22"=w419, "Connector1/DIO23"=w418, "Connector1/DIO24"=w417, "Connector1/DIO25"=w416, "Connector1/DIO26"=w415, "Connector1/DIO27"=w414) -> ()  [unwired: 22 in, 22 out]
              }
              frame #2 {
                # "wait and then apply write signal"
                n244 = call "Wait2"("Count(Ticks)"=u8 40 ("DO Delay 1 (Ticks)")) -> ()  [unwired: 1 out]
              }
              frame #3 {
                # "sending bit low writes data to board buffer"
                n245 = xnode "FPGA I/O Node"("Connector1/DIO15"=FALSE) -> ()  [unwired: 1 in, 1 out]
              }
              frame #4 {
                # "wait then return write signal"
                n246 = call "Wait3"("Count(Ticks)"=u8 40 ("DO Delay 2 (Ticks)")) -> ()  [unwired: 1 out]
              }
              frame #5 {
                # "sending bit high makes ready to\nwrite more data"
                n247 = xnode "FPGA I/O Node"("Connector1/DIO15"=TRUE) -> ()  [unwired: 1 in, 1 out]
              }
            }
          }
        }
      }
    }
  }
  n248 = To Unsigned Long Integer(number=w2) -> (unsigned 32bit integer=w4:u32)
  n249 = while "APD 1 Counter" {
    tunnel: w2 -> [_]
    stop <- FALSE stop-if-true
    n250 = flat-sequence {
      frame #0 {
        n251 = xnode "FPGA I/O Method Node"("FPGA I/O In"=refnum<k21> "Connector0/DIO0" ("APD 1 DO"), "Timeout"=-1) -> ()  [unwired: 2 out]
      }
      frame #1 {
        n252 = local read "APD1 out state"() -> (w471:bool)
        n253 = case shown="False" w471 {
          frame False {
            n254 = local read "APD 1 Counts 0"() -> (w473:u32)
            n255 = Increment(x=w473) -> (x+1=→"APD 1 Counts 0":u32)
          }
          frame True {
            n256 = local read "APD 1 Counts 1"() -> (w475:u32)
            n257 = Increment(x=w475) -> (x+1=→"APD 1 Counts 1":u32)
          }
        }
      }
    }
  }
  n258 = while "APD 2 Counter" {
    tunnel: w2 -> [_]
    stop <- FALSE stop-if-true
    n259 = flat-sequence {
      frame #0 {
        n260 = xnode "FPGA I/O Method Node"("FPGA I/O In"=refnum<k21> "Connector0/DIO1" ("APD 2 DO"), "Timeout"=-1) -> ()  [unwired: 2 out]
      }
      frame #1 {
        n261 = local read "APD2 out state"() -> (w479:bool)
        n262 = case shown="False" w479 {
          frame False {
            n263 = local read "APD 2 Counts 0"() -> (w481:u32)
            n264 = Increment(x=w481) -> (x+1=→"APD 2 Counts 0":u32)
          }
          frame True {
            n265 = local read "APD 2 Counts 1"() -> (w483:u32)
            n266 = Increment(x=w483) -> (x+1=→"APD 2 Counts 1":u32)
          }
        }
      }
    }
  }
  n267 = while "APD 2 Gating" {
    shift-right: [w487] -> _
    shift-left: w2 -> [w492]
    shift-right: [w486] -> _
    shift-left: w3 -> [w484]
    stop <- FALSE stop-if-true
    n268 = flat-sequence {
      tunnel: w492 -> [w495]
      tunnel: [w496] -> w490
      tunnel: [w495] -> w488
      tunnel: [w494] -> w485
      tunnel: w484 -> [w494]
      tunnel: [w499] -> w491
      tunnel: w490 -> [w499]
      tunnel: [w498] -> w489
      tunnel: w488 -> [w498]
      tunnel: w485 -> [w497]
      tunnel: [w517] -> w487
      tunnel: w491 -> [w528]
      tunnel: w489 -> [w526]
      tunnel: [w521] -> w486
      frame #0 {
        n269 = call "Loop Timer8"("Count(Ticks)"=w495) -> ("Tick Count(Ticks)"=w496:u16)
      }
      frame #1 {
        # "Signal is then sent through \na transistor before APD"
        n270 = xnode "FPGA I/O Node"("Connector0/DIO8"=w497) -> ()  [unwired: 1 in, 1 out]
      }
      frame #2 {
        n271 = local read "APD Gate ON Count"() -> (w510:u16)
        n272 = local read "APD Gate OFF Count"() -> (w509:u16)
        n273 = feedback #16(TRUE) -> (w523:bool)
        n274 = feedback-in #17(w528) -> ()
        n275 = feedback #17(w528) -> (w511:u16)
        n276 = Not(x=w523) -> (.not. x?=w520:bool)
        n277 = feedback-in #16(w520) -> ()
        n278 = Subtract(x=w528, y=w511) -> (x-y=w527:u16)
        n279 = Select(t=w510, s=w520, f=w509) -> (s? t:f=w525:u16)
        n280 = Subtract(x=w527, y=w526) -> (x-y=w502:u16)
        n281 = Subtract(x=w525, y=w502) -> (x-y=w516:u16)
        n282 = Number To Boolean Array(number=w502) -> (Boolean array=w501:bool[])
        n283 = Or Array Elements(Boolean array=w501) -> (logical OR=w500:bool)
        n284 = Boolean To (0,1)(Boolean="+ phase (APD 2 Gate)") -> (0, 1=w514:i16)
        n285 = Multiply(x=w514, y="Phase count adjustment (APD 2 Gate)") -> (x*y=w512:i16)
        n286 = Boolean To (0,1)(Boolean=w500) -> (0, 1=w507:i16)
        n287 = Add(x=w516, y=w512) -> (x+y=w517:u16)
        n288 = To Unsigned Byte Integer(number=w507) -> (unsigned 8bit integer=w504:u8)
        n289 = feedback #18(i16 0) -> (w519:i16)
        n290 = Subtract(x=w519, y=w512) -> (x-y=w518:i16)
        "APD 2 Gate Relative Phase" <- w518
        n291 = feedback-in #18(w518) -> ()
        n292 = feedback #19(u8 0) -> (w505:u8)
        n293 = Add(x=w504, y=w505) -> (x+y=w503:u8)
        "APD 2 Gate Late Counter" <- w503
        n294 = feedback-in #19(w503) -> ()
        n295 = local read "APD Gate Operating Mode"() -> (w508:u8)
        n296 = case shown="2" w508 {
          tunnel: [TRUE FALSE w534] -> w521
          tunnel: w523 -> [_ _ w532]
          frame 0, Default {
          }
          frame 1 {
          }
          frame 2 {
            n297 = local read "Invert APD Gate"() -> (w531:bool)
            n298 = Not(x=w532) -> (.not. x?=w533:bool)
            n299 = Select(t=w533, s=w531, f=w532) -> (s? t:f=w534:bool)
          }
        }
      }
    }
  }
  n300 = while "DAQ AI set 1" {
    shift-right: [w535] -> _
    shift-left: w2 -> [w540]
    stop <- FALSE stop-if-true
    n301 = flat-sequence {
      tunnel: w540 -> [w550]
      tunnel: [w551] -> w538
      tunnel: [w550] -> w537
      tunnel: [w561] -> w548
      tunnel: [w560] -> w547
      tunnel: [w559] -> w546
      tunnel: [w558] -> w545
      tunnel: [w557] -> w544
      tunnel: [w556] -> w543
      tunnel: [w555] -> w542
      tunnel: [w554] -> w541
      tunnel: [w553] -> w539
      tunnel: w538 -> [w553]
      tunnel: w537 -> [w552]
      tunnel: [w552] -> w536
      tunnel: [w590] -> w535
      tunnel: w548 -> [w617]
      tunnel: w547 -> [w582]
      tunnel: w546 -> [w583]
      tunnel: w545 -> [w616]
      tunnel: w544 -> [w606]
      tunnel: w543 -> [w605]
      tunnel: w542 -> [w604]
      tunnel: w541 -> [w603]
      tunnel: w539 -> [w600]
      tunnel: w536 -> [w597]
      frame #0 {
        n302 = call "Loop Timer3"("Count(Ticks)"=w550) -> ("Tick Count(Ticks)"=w551:u16)
      }
      frame #1 {
        n303 = xnode "FPGA I/O Node"("Connector1/DIO31"=TRUE ("Connector1/DIO33")) -> ("Connector0/AI0"=w561:i16, "Connector0/AI1"=w560:i16, "Connector0/AI2"=w559:i16, "Connector0/AI3"=w558:i16, "Connector0/AI4"=w557:i16, "Connector0/AI5"=w556:i16, "Connector0/AI6"=w555:i16, "Connector0/AI7"=w554:i16)  [unwired: 9 in, 9 out]
      }
      frame #2 {
        w586 = FALSE ("AI to FIFO")
        # "Adjust phase after data acquired if button pressed"
        n304 = feedback #20(i16 1) -> (w609:i16)
        n305 = Increment(x=w609) -> (x+1=w615:i16)
        n306 = Scale By Power Of 2(n="AI1 X Scale", x=w582) -> (x*2^n=w580:i16)
        n307 = Greater?(x=w615, y="N of AI1 Int Acq Sets") -> (0:w612:bool)
        n308 = Select(t=i16 1, s=w612, f=w615) -> (s? t:f=w614:i16)
        n309 = feedback-in #20(w614) -> ()
        n310 = Divide(x=w580, y=w583) -> (x/y=w579:fxp<+/-,16,1>)
        n311 = feedback #21(w586) -> (w584:bool)
        n312 = feedback #22(w586) -> (w602:bool)
        n313 = case shown="2" w609 {
          tunnel: w583 -> [w640 w647 _]
          tunnel: ["Set 1" "Set 2" "Set 3"] -> w607
          tunnel: ["AI to FIFO" w649 w654] -> w601
          tunnel: w602 -> [_ w649 w654]
          tunnel: ["Trap Pos to FIFO" w648 w653] -> w585
          tunnel: w584 -> [_ w648 w653]
          tunnel: w579 -> [w639 w646 _]
          tunnel: [w638 w644 FALSE] -> w566
          tunnel: [w637 w645 u64 0 ("BD1 Frequency Out 2")] -> w565
          frame 1, Default {
            n314 = local read "BD1 Frequency Out 1"() -> (w637:u64)
            n315 = Compound Arithmetic op=AND("Trap Pos to FIFO", "Set 1", "AI to FIFO") -> (w638:bool)
            "AI2 Y Sum Set 1" <- w640
            "AI1 X Set 1" <- w639
          }
          frame 2 {
            n316 = local read "BD1 Frequency Out 2"() -> (w645:u64)
            n317 = Compound Arithmetic op=AND(w648, "Set 2", w649) -> (w644:bool)
            "AI2 Y Sum Set 2" <- w647
            "AI1 X Set 2" <- w646
          }
          frame 3 {
          }
        }
        n318 = And(x=w607, y=w601) -> (x .and. y?=w608:bool)
        n319 = case shown="True" w608 {
          tunnel: w617 -> [_ w668]
          tunnel: w582 -> [_ w667]
          tunnel: w583 -> [_ w666]
          tunnel: w616 -> [_ w665]
          tunnel: w606 -> [_ w664]
          tunnel: w605 -> [_ w663]
          tunnel: w604 -> [_ w662]
          tunnel: w603 -> [_ w661]
          tunnel: 0 ("DMA buffer timeout") -> [_ w670]
          frame False {
          }
          frame True {
            n320 = Build Array(w668, w667, w666, w665, w664, w663, w662, w661) -> (w669:i16[])
            n321 = for {
              tunnel: w669 -> [w672] mode=indexing
              tunnel: w670 -> [w673]
              tunnel: [w671] -> w659 mode=indexing
              n322 = xnode ("FIFO Write")("Element"=w672, "Timeout"=w673) -> ("Timed Out?"=w671:bool)  [unwired: 1 in, 1 out]
            }
            n323 = Or Array Elements(Boolean array=w659) -> (logical OR=w656:bool)
            n324 = Boolean To (0,1)(Boolean=w656) -> (0, 1=w658:i16)
            n325 = feedback #23(u16 0) -> (w657:u16)
            n326 = Add(x=w658, y=w657) -> (x+y=w655:u16)
            "Trap AI FIFO Timeout" <- w655
            n327 = feedback-in #23(w655) -> ()
          }
        }
        n328 = feedback-in #21(w585) -> ()
        n329 = feedback-in #22(w601) -> ()
        n330 = case shown="True" w566 {
          tunnel: w565 -> [_ w623]
          tunnel: [u8 0 w620] -> w564
          frame False {
          }
          frame True {
            n331 = Split Number(x=w623) -> (hi(x)=w624:u32, lo(x)=w625:u32)
            n332 = Split Number(x=w624) -> (lo(x)=w626:u16)  [unwired: 1 out]
            n333 = Split Number(x=w625) -> (hi(x)=w627:u16, lo(x)=w628:u16)
            n334 = Build Array "BD 1 nu Stack"(w626, w627, w628) -> (w622:u16[])
            n335 = for {
              tunnel: w622 -> [w635] mode=indexing
              shift-right: [w631] -> w620
              shift-left: u8 0 -> [w632]
              n336 = xnode ("FIFO Method Node")("Element"=w635, "Timeout"="Trap FIFO Set Timeout") -> ("Timed Out?"=w634:bool)  [unwired: 1 in, 1 out]
              n337 = Boolean To (0,1)(Boolean=w634) -> (0, 1=w633:i16)
              n338 = To Unsigned Byte Integer(number=w633) -> (unsigned 8bit integer=w630:u8)
              n339 = Add(x=w630, y=w632) -> (x+y=w631:u8)
            }
          }
        }
        n340 = To Unsigned Word Integer(number=w564) -> (unsigned 16bit integer=w563:u16)
        n341 = feedback #24(u16 0) -> (w577:u16)
        n342 = Add(x=w563, y=w577) -> (x+y=w576:u16)
        "Trap Pos FIFO Timeout" <- w576
        n343 = feedback-in #24(w576) -> ()
        n344 = feedback-in #25(w600) -> ()
        n345 = feedback #25(w600) -> (w599:u16)
        n346 = Subtract(x=w600, y=w599) -> (x-y=w598:u16)
        n347 = xnode "FPGA I/O Node"("Connector1/DIO31"=FALSE ("Connector1/DIO34")) -> ()  [unwired: 1 in, 1 out]
        n348 = Subtract(x=w598, y=w597) -> (x-y=w568:u16)
        n349 = Boolean To (0,1)(Boolean="+ phase") -> (0, 1=w593:i16)
        n350 = Multiply(x=w593, y="Phase count adjustment") -> (x*y=w587:i16)
        n351 = Subtract(x="ai count", y=w568) -> (x-y=w591:u16)
        n352 = Number To Boolean Array(number=w568) -> (Boolean array=w569:bool[])
        n353 = feedback #26(i16 0) -> (w589:i16)
        n354 = Add(x=w591, y=w587) -> (x+y=w590:u16)
        n355 = Subtract(x=w589, y=w587) -> (x-y=w588:i16)
        "Relative phase" <- w588
        n356 = feedback-in #26(w588) -> ()
        n357 = Or Array Elements(Boolean array=w569) -> (logical OR=w567:bool)
        n358 = Boolean To (0,1)(Boolean=w567) -> (0, 1=w574:i16)
        n359 = To Unsigned Byte Integer(number=w574) -> (unsigned 8bit integer=w571:u8)
        n360 = feedback #27(u8 0) -> (w572:u8)
        n361 = Add(x=w571, y=w572) -> (x+y=w570:u8)
        "AI Late Counter" <- w570
        n362 = feedback-in #27(w570) -> ()
      }
    }
  }
  n363 = while "MCL stage control" {
    shift-right: [w686] -> _
    shift-left: w2 -> [w689]
    shift-right: [w679] -> _
    shift-left: w9 -> [w676]
    shift-right: [w678] -> _
    shift-left: w8 -> [w674]
    stop <- FALSE stop-if-true
    n364 = flat-sequence {
      tunnel: w689 -> [w693]
      tunnel: [w694] -> w685
      tunnel: [w693] -> w683
      tunnel: [w692] -> w677
      tunnel: w676 -> [w692]
      tunnel: [w691] -> w675
      tunnel: w674 -> [w691]
      tunnel: w685 -> [w698]
      tunnel: [w698] -> w684
      tunnel: w683 -> [w697]
      tunnel: [w697] -> w682
      tunnel: w677 -> [w696]
      tunnel: w675 -> [w695]
      tunnel: w684 -> [w706]
      tunnel: w682 -> [w705]
      tunnel: [w706] -> w688
      tunnel: [w705] -> w687
      tunnel: [w704] -> w681
      tunnel: [w703] -> w680
      tunnel: [w778] -> w686
      tunnel: w688 -> [w785]
      tunnel: w687 -> [w782]
      tunnel: w681 -> [w780]
      tunnel: w680 -> [w779]
      tunnel: [w780] -> w679
      tunnel: [w779] -> w678
      frame #0 {
        n365 = call "Loop Timer5"("Count(Ticks)"=w693) -> ("Tick Count(Ticks)"=w694:u32)
      }
      frame #1 {
        n366 = xnode "FPGA I/O Node"("Connector0/AO1"=w696, "Connector0/AO2"=w695) -> ()  [unwired: 2 in, 2 out]
      }
      frame #2 {
        n367 = local read "Scanning MCL"() -> (w718:bool)
        n368 = Or(x=w718, y="Start scan (MCL)") -> (x .or. y?=w713:bool)
        n369 = Not(x="Abort scan (MCL)") -> (.not. x?=w711:bool)
        n370 = And(x=w711, y=w713) -> (x .and. y?=w710:bool)
        n371 = case "Raster scan" shown="True" w710 {
          tunnel: [w719 w762] -> w715
          tunnel: "Start scan (MCL)" -> [_ w747]
          tunnel: [w719 w723] -> w699
          frame False {
            w719 = i16 0
            n372 = local write "Scanning MCL"(FALSE ("scanning")) -> ()
          }
          frame True {
            w733 = i16 0
            w732 = u64 0
            # "scan incr."
            # "freq. incr. mult."
            # "count steps"
            # "count number of cycles"
            n373 = feedback #28(w732) -> (w759:u64)
            n374 = Select(t=w732, s=w747, f=w759) -> (s? t:f=w761:u64)
            n375 = Increment(x=w761) -> (x+1=w758:u64)
            n376 = Greater?(x="Cycles per step (MCL)", y=w758) -> (0:w742:bool)
            n377 = Select(t=w758, s=w742, f=w732) -> (s? t:f=w757:u64)
            n378 = feedback-in #28(w757) -> ()
            n379 = feedback #29(w732) -> (w756:u64)
            n380 = Select(t=w732, s=w747, f=w756) -> (s? t:f=w751:u64)
            n381 = Increment(x=w751) -> (x+1=w755:u64)
            n382 = Add(x="Scan steps (MCL)", y="Scan steps (MCL)") -> (x+y=w754:u64)
            n383 = Select(t=w751, s=w742, f=w755) -> (s? t:f=w737:u64)
            n384 = Greater?(x=w754, y=w737) -> (0:w736:bool)
            n385 = Select(t=w737, s=w736, f=w732) -> (s? t:f=w752:u64)
            n386 = feedback-in #29(w752) -> ()
            n387 = Equal?(x="Scan steps (MCL)", y=w737) -> (x = y?=w741:bool)
            n388 = Greater?(x="Scan steps (MCL)", y=w751) -> (0:w750:bool)
            n389 = feedback #30(w733) -> (w753:i16)
            n390 = Select(t=w733, s=w747, f=w753) -> (s? t:f=w739:i16)
            n391 = Increment(x=w739) -> (x+1=w749:i16)
            n392 = Decrement(x=w739) -> (x-1=w748:i16)
            n393 = Select(t=w749, s=w750, f=w748) -> (s? t:f=w740:i16)
            n394 = Select(t=w739, s=w741, f=w740) -> (s? t:f=w738:i16)
            n395 = Select(t=w739, s=w742, f=w738) -> (s? t:f=w734:i16)
            n396 = Select(t=w734, s=w736, f=w733) -> (s? t:f=w735:i16)
            n397 = feedback-in #30(w735) -> ()
            n398 = feedback #31(w732) -> (w746:u64)
            n399 = Select(t=w732, s=w747, f=w746) -> (s? t:f=w721:u64)
            n400 = Increment(x=w721) -> (x+1=w743:u64)
            n401 = Select(t=w721, s=w736, f=w743) -> (s? t:f=w722:u64)
            n402 = Greater?(x="Number of scans (MCL)", y=w722) -> (0:w729:bool)
            n403 = Multiply(x="Scan freq.  increment (MCL)", y=w739) -> (x*y=w762:i16)
            n404 = Select(t=TRUE, s="Cont. Scan (MCL)", f=w729) -> (s? t:f=w728:bool)
            "Scanning MCL" <- w728
            n405 = Select(t=w722, s=w728, f=w732) -> (s? t:f=w744:u64)
            n406 = feedback-in #31(w744) -> ()
            n407 = Increment(x=w722) -> (x+1=→"Scan I (MCL)":u64)
            n408 = To Word Integer(number=w721) -> (16bit integer=w724:i16)
            n409 = Multiply(x=w724, y="Scan freq.  increment (MCL)") -> (x*y=w723:i16)
          }
        }
        n410 = Select(t=w699, s="1D or 2D Scan?", f=i16 0) -> (s? t:f=w700:i16)
        n411 = Select(t=w700, s="MCL Scan Axis", f=w715) -> (s? t:f=w714:i16)
        n412 = Select(t=w715, s="MCL Scan Axis", f=w700) -> (s? t:f=w716:i16)
        n413 = Add(x=w714, y="AO2") -> (x+y=w703:i16)
        n414 = Add(x="AO1", y=w716) -> (x+y=w704:i16)
      }
      frame #3 {
        n415 = feedback-in #32(w785) -> ()
        n416 = feedback #32(w785) -> (w784:u32)
        n417 = Boolean To (0,1)(Boolean="+ phase (MCL)") -> (0, 1=w776:i16)
        n418 = Subtract(x=w785, y=w784) -> (x-y=w783:u32)
        n419 = Multiply(x=w776, y="Phase count adjustment (MCL)") -> (x*y=w772:i16)
        n420 = Subtract(x=w783, y=w782) -> (x-y=w764:u32)
        n421 = Subtract(x="MCL count", y=w764) -> (x-y=w774:u32)
        n422 = feedback #33(i16 0) -> (w773:i16)
        n423 = Subtract(x=w773, y=w772) -> (x-y=w771:i16)
        "MCL Relative Phase" <- w771
        n424 = feedback-in #33(w771) -> ()
        n425 = Number To Boolean Array(number=w764) -> (Boolean array=w765:bool[])
        n426 = Or Array Elements(Boolean array=w765) -> (logical OR=w763:bool)
        n427 = Boolean To (0,1)(Boolean=w763) -> (0, 1=w770:i16)
        n428 = Add(x=w774, y=w772) -> (x+y=w778:u32)
        n429 = To Unsigned Byte Integer(number=w770) -> (unsigned 8bit integer=w767:u8)
        n430 = feedback #34(u8 0) -> (w768:u8)
        n431 = Add(x=w767, y=w768) -> (x+y=w766:u8)
        "MCL Late Counter" <- w766
        n432 = feedback-in #34(w766) -> ()
      }
    }
  }
  n433 = while "APD 1 Gating" {
    shift-right: [w790] -> _
    shift-left: w2 -> [w795]
    shift-right: [w789] -> _
    shift-left: w3 -> [w787]
    stop <- FALSE stop-if-true
    n434 = flat-sequence {
      tunnel: w795 -> [w798]
      tunnel: [w799] -> w793
      tunnel: [w798] -> w791
      tunnel: [w797] -> w788
      tunnel: w787 -> [w797]
      tunnel: [w802] -> w794
      tunnel: w793 -> [w802]
      tunnel: [w801] -> w792
      tunnel: w791 -> [w801]
      tunnel: w788 -> [w800]
      tunnel: [w816] -> w790
      tunnel: w794 -> [w831]
      tunnel: w792 -> [w828]
      tunnel: [w820] -> w789
      frame #0 {
        n435 = call "Loop Timer7"("Count(Ticks)"=w798) -> ("Tick Count(Ticks)"=w799:u16)
      }
      frame #1 {
        # "Signal is then sent through \na transistor before APD"
        n436 = xnode "FPGA I/O Node"("Connector0/DIO4"=w800) -> ()  [unwired: 1 in, 1 out]
      }
      frame #2 {
        n437 = feedback #35(TRUE) -> (w823:bool)
        n438 = feedback-in #36(w831) -> ()
        n439 = feedback #36(w831) -> (w830:u16)
        n440 = Not(x=w823) -> (.not. x?=w819:bool)
        n441 = feedback-in #35(w819) -> ()
        n442 = Subtract(x=w831, y=w830) -> (x-y=w829:u16)
        n443 = Select(t="APD Gate ON Count", s=w819, f="APD Gate OFF Count") -> (s? t:f=w825:u16)
        n444 = Subtract(x=w829, y=w828) -> (x-y=w804:u16)
        n445 = Subtract(x=w825, y=w804) -> (x-y=w815:u16)
        n446 = Number To Boolean Array(number=w804) -> (Boolean array=w805:bool[])
        n447 = Or Array Elements(Boolean array=w805) -> (logical OR=w803:bool)
        n448 = Boolean To (0,1)(Boolean="+ phase (APD 1 Gate)") -> (0, 1=w813:i16)
        n449 = Boolean To (0,1)(Boolean=w803) -> (0, 1=w810:i16)
        n450 = Multiply(x=w813, y="Phase count adjustment (APD 1 Gate)") -> (x*y=w811:i16)
        n451 = To Unsigned Byte Integer(number=w810) -> (unsigned 8bit integer=w807:u8)
        n452 = Add(x=w815, y=w811) -> (x+y=w816:u16)
        n453 = feedback #37(i16 0) -> (w818:i16)
        n454 = Subtract(x=w818, y=w811) -> (x-y=w817:i16)
        "APD 1 Gate Relative Phase" <- w817
        n455 = feedback-in #37(w817) -> ()
        n456 = feedback #38(u8 0) -> (w808:u8)
        n457 = Add(x=w807, y=w808) -> (x+y=w806:u8)
        "APD 1 Gate Late Counter" <- w806
        n458 = feedback-in #38(w806) -> ()
        n459 = case shown="2" "APD Gate Operating Mode" {
          tunnel: [TRUE FALSE w837] -> w820
          tunnel: w823 -> [_ _ w834]
          frame 0, Default {
          }
          frame 1 {
          }
          frame 2 {
            n460 = Not(x=w834) -> (.not. x?=w836:bool)
            n461 = Select(t=w836, s="Invert APD Gate", f=w834) -> (s? t:f=w837:bool)
          }
        }
      }
    }
  }
  n462 = while "Control APD data integration - stream to host" {
    shift-right: [w841] -> _
    shift-left: w4 -> [w846]
    stop <- FALSE stop-if-true
    n463 = flat-sequence {
      tunnel: w846 -> [w848]
      tunnel: [w849] -> w844
      tunnel: [w848] -> w842
      tunnel: [w859] -> w845
      tunnel: w844 -> [w859]
      tunnel: [w858] -> w843
      tunnel: w842 -> [w858]
      tunnel: [w857] -> w840
      tunnel: [w856] -> w839
      tunnel: [w850] -> w838
      tunnel: [w901] -> w841
      tunnel: w845 -> [w911]
      tunnel: w843 -> [w908]
      tunnel: w840 -> [w894]
      tunnel: w839 -> [w893]
      tunnel: w838 -> [w881]
      frame #0 {
        n464 = call "Loop Timer6"("Count(Ticks)"=w848) -> ("Tick Count(Ticks)"=w849:u32)
      }
      frame #1 {
        n465 = flat-sequence {
          tunnel: [w861] -> w855
          tunnel: w855 -> [w864]
          tunnel: [w868] -> w854
          tunnel: [w867] -> w853
          tunnel: [w864] -> w852
          tunnel: [w863] -> w851
          tunnel: [w875] -> w856
          tunnel: [w876] -> w857
          tunnel: w854 -> [w876]
          tunnel: w853 -> [w875]
          tunnel: w852 -> [w874]
          tunnel: w851 -> [w873]
          tunnel: [w873] -> w850
          frame #0 {
            # "use separate variable so each APD won't\nhave to wait to read"
            n466 = feedback #39(FALSE) -> (w860:bool)
            "APD1 out state" <- w860
            "APD2 out state" <- w860
            "APD3 out state" <- w860
            n467 = Not(x=w860) -> (.not. x?=w861:bool)
            n468 = feedback-in #39(w861) -> ()
          }
          frame #1 {
            n469 = local read "APD 3 Counts 1"() -> (w866:u32)
            n470 = local read "APD 3 Counts 0"() -> (w865:u32)
            n471 = local read "APD 1 Counts 1"() -> (w872:u32)
            n472 = local read "APD 1 Counts 0"() -> (w871:u32)
            n473 = local read "APD 2 Counts 1"() -> (w870:u32)
            n474 = local read "APD 2 Counts 0"() -> (w869:u32)
            n475 = Select(t=w866, s=w864, f=w865) -> (s? t:f=w863:u32)
            n476 = Select(t=w872, s=w864, f=w871) -> (s? t:f=w868:u32)
            n477 = Select(t=w870, s=w864, f=w869) -> (s? t:f=w867:u32)
          }
          frame #2 {
            n478 = case shown="False" w874 {
              frame False {
                w877 = u32 0 ("APD 1 Counts 0")
                n479 = local write "APD 1 Counts 0"(w877) -> ()
                n480 = local write "APD 2 Counts 0"(w877) -> ()
                n481 = local write "APD 3 Counts 0"(w877) -> ()
              }
              frame True {
                w878 = u32 0 ("APD 1 Counts 1")
                n482 = local write "APD 1 Counts 1"(w878) -> ()
                n483 = local write "APD 2 Counts 1"(w878) -> ()
                n484 = local write "APD 3 Counts 1"(w878) -> ()
              }
            }
          }
        }
      }
      frame #2 {
        n485 = feedback-in #40(w911) -> ()
        n486 = feedback #40(w911) -> (w910:u32)
        n487 = Subtract(x=w911, y=w910) -> (x-y=w909:u32)
        n488 = Subtract(x=w909, y=w908) -> (x-y=w886:u32)
        n489 = case shown="True" "APD to FIFO" {
          tunnel: w894 -> [_ w916]
          tunnel: w893 -> [_ w914]
          tunnel: w881 -> [_ w912]
          frame False {
          }
          frame True {
            n490 = flat-sequence {
              tunnel: 0 ("Timeout") -> [w918]
              tunnel: w916 -> [w919]
              tunnel: [w918] -> w915
              tunnel: w915 -> [w920]
              tunnel: w914 -> [w921]
              tunnel: [w920] -> w913
              tunnel: w913 -> [w923]
              tunnel: w912 -> [w922]
              frame #0 {
                n491 = xnode ("FIFO Write")("Element"=w919, "Timeout"=w918) -> ()  [unwired: 1 in, 2 out]
              }
              frame #1 {
                n492 = xnode ("FIFO Write")("Element"=w921, "Timeout"=w920) -> ()  [unwired: 1 in, 2 out]
              }
              frame #2 {
                n493 = xnode ("FIFO Write")("Element"=w922, "Timeout"=w923) -> ()  [unwired: 1 in, 2 out]
              }
            }
          }
        }
        n494 = Subtract(x="APD Acq Rate Count", y=w886) -> (x-y=w902:u32)
        n495 = Number To Boolean Array(number=w886) -> (Boolean array=w887:bool[])
        n496 = Or Array Elements(Boolean array=w887) -> (logical OR=w885:bool)
        n497 = Boolean To (0,1)(Boolean=w885) -> (0, 1=w892:i16)
        n498 = To Unsigned Byte Integer(number=w892) -> (unsigned 8bit integer=w889:u8)
        n499 = feedback #41(u8 0) -> (w890:u8)
        n500 = Add(x=w889, y=w890) -> (x+y=w888:u8)
        "APD Acq Late Counter" <- w888
        n501 = feedback-in #41(w888) -> ()
        n502 = Boolean To (0,1)(Boolean="+ phase (APD Acq)") -> (0, 1=w898:i16)
        n503 = Multiply(x=w898, y="Phase Count Adjustment (APD Acq)") -> (x*y=w895:i16)
        n504 = Add(x=w902, y=w895) -> (x+y=w901:u32)
        n505 = feedback #42(i16 0) -> (w900:i16)
        n506 = Subtract(x=w900, y=w895) -> (x-y=w897:i16)
        "APD Acq Relative Phase" <- w897
        n507 = feedback-in #42(w897) -> ()
        n508 = To Word Integer(number=w894) -> (16bit integer=w903:i16)
        n509 = To Word Integer(number=w881) -> (16bit integer=w882:i16)
        n510 = To Word Integer(number=w893) -> (16bit integer=w904:i16)
        n511 = Multiply(x="APD AO scale factor", y=w904) -> (x*y=w883:i16)
        n512 = Multiply(x="APD AO scale factor", y=w882) -> (x*y=w879:i16)
        n513 = Multiply(x="APD AO scale factor", y=w903) -> (x*y=w884:i16)
        n514 = xnode "FPGA I/O Node"("Connector0/AO5"=w884, "Connector0/AO7"=w883, "Connector0/AO6"=w879) -> ()  [unwired: 3 in, 3 out]
      }
    }
  }
  n515 = while "532 nm green fluorescent laser interlacing (DO to IA 532 nm AOM ME amp)." {
    shift-right: [w927] -> _
    shift-left: w2 -> [w932]
    shift-right: [w926] -> _
    shift-left: FALSE -> [w924]
    stop <- FALSE stop-if-true
    n516 = flat-sequence {
      tunnel: w932 -> [w935]
      tunnel: [w936] -> w930
      tunnel: [w935] -> w928
      tunnel: [w934] -> w925
      tunnel: w924 -> [w934]
      tunnel: [w939] -> w931
      tunnel: w930 -> [w939]
      tunnel: [w938] -> w929
      tunnel: w928 -> [w938]
      tunnel: w925 -> [w937]
      tunnel: [w948] -> w927
      tunnel: w931 -> [w968]
      tunnel: w929 -> [w965]
      tunnel: [w957] -> w926
      frame #0 {
        n517 = call "Loop Timer4"("Count(Ticks)"=w935) -> ("Tick Count(Ticks)"=w936:u16)
      }
      frame #1 {
        # "Then to PRL 440 amp"
        n518 = xnode "FPGA I/O Node"("Connector1/DIO39"=w937) -> ()  [unwired: 1 in, 1 out]
      }
      frame #2 {
        n519 = feedback-in #43(w968) -> ()
        n520 = feedback #43(w968) -> (w967:u16)
        n521 = Subtract(x=w968, y=w967) -> (x-y=w966:u16)
        n522 = Subtract(x=w966, y=w965) -> (x-y=w941:u16)
        n523 = Number To Boolean Array(number=w941) -> (Boolean array=w942:bool[])
        n524 = Or Array Elements(Boolean array=w942) -> (logical OR=w940:bool)
        n525 = Boolean To (0,1)(Boolean="+ phase (GI)") -> (0, 1=w953:i16)
        n526 = Multiply(x=w953, y="Phase count adjustment (GI)") -> (x*y=w950:i16)
        n527 = Boolean To (0,1)(Boolean=w940) -> (0, 1=w947:i16)
        n528 = To Unsigned Byte Integer(number=w947) -> (unsigned 8bit integer=w944:u8)
        n529 = feedback #44(i16 0) -> (w951:i16)
        n530 = feedback #45(u8 0) -> (w945:u8)
        n531 = Add(x=w944, y=w945) -> (x+y=w943:u8)
        "GI Late Counter" <- w943
        n532 = feedback-in #45(w943) -> ()
        n533 = Subtract(x=w951, y=w950) -> (x-y=w949:i16)
        "GI Relative phase" <- w949
        n534 = feedback-in #44(w949) -> ()
        n535 = feedback #46(TRUE) -> (w960:bool)
        n536 = case shown="2" "Operating Mode" {
          tunnel: [TRUE FALSE w974] -> w957
          tunnel: w960 -> [_ _ w971]
          frame 0, Default {
          }
          frame 1 {
          }
          frame 2 {
            n537 = Not(x=w971) -> (.not. x?=w973:bool)
            n538 = Select(t=w973, s="Invert GI", f=w971) -> (s? t:f=w974:bool)
          }
        }
        n539 = Not(x=w960) -> (.not. x?=w956:bool)
        n540 = Select(t="Green interlace ON count", s=w956, f="Green interlace OFF count") -> (s? t:f=w962:u16)
        n541 = Subtract(x=w962, y=w941) -> (x-y=w954:u16)
        n542 = Add(x=w954, y=w950) -> (x+y=w948:u16)
        n543 = feedback-in #46(w956) -> ()
      }
    }
  }
  n544 = while "Green fluorescent laser interlacing (Current to IA 532 nm AOM ME amp)." {
    shift-right: [w980] -> _
    shift-left: w2 -> [w983]
    shift-right: [w977] -> _
    shift-left: u16 0 -> [w975]
    stop <- FALSE stop-if-true
    n545 = flat-sequence {
      tunnel: w983 -> [w986]
      tunnel: [w987] -> w982
      tunnel: [w986] -> w981
      tunnel: [w985] -> w976
      tunnel: w975 -> [w985]
      tunnel: [w990] -> w979
      tunnel: w982 -> [w990]
      tunnel: [w989] -> w978
      tunnel: w981 -> [w989]
      tunnel: w976 -> [w988]
      tunnel: [w999] -> w980
      tunnel: [w1016] -> w977
      tunnel: w979 -> [w1029]
      tunnel: w978 -> [w1026]
      frame #0 {
        n546 = call "Loop Timer10"("Count(Ticks)"=w986) -> ("Tick Count(Ticks)"=w987:u16)
      }
      frame #1 {
        n547 = xnode "FPGA I/O Node"("Chassis2/Mod4/AO0"=w988) -> ()  [unwired: 1 in, 1 out]
      }
      frame #2 {
        n548 = Subtract(x="Green interlace OFF count 2", y="Green int current ON count adj") -> (x-y=w1008:u16)
        n549 = feedback-in #47(w1029) -> ()
        n550 = feedback #47(w1029) -> (w1028:u16)
        n551 = Add(x="Green int current ON count adj", y="Green interlace ON count 2") -> (x+y=w1009:u16)
        n552 = Subtract(x=w1029, y=w1028) -> (x-y=w1027:u16)
        n553 = Subtract(x=w1027, y=w1026) -> (x-y=w992:u16)
        n554 = Number To Boolean Array(number=w992) -> (Boolean array=w993:bool[])
        n555 = Boolean To (0,1)(Boolean="+ phase (GI) 2") -> (0, 1=w1005:i16)
        n556 = Or Array Elements(Boolean array=w993) -> (logical OR=w991:bool)
        n557 = Boolean To (0,1)(Boolean=w991) -> (0, 1=w998:i16)
        n558 = Multiply(x=w1005, y="Phase count adjustment (GI) 2") -> (x*y=w1001:i16)
        n559 = To Unsigned Byte Integer(number=w998) -> (unsigned 8bit integer=w994:u8)
        n560 = feedback #48(u8 0) -> (w996:u8)
        n561 = Add(x=w994, y=w996) -> (x+y=w995:u8)
        "GI Late Counter 2" <- w995
        n562 = feedback-in #48(w995) -> ()
        n563 = feedback #49(i16 0) -> (w1002:i16)
        n564 = Subtract(x=w1002, y=w1001) -> (x-y=w1000:i16)
        "GI Relative phase 2" <- w1000
        n565 = feedback-in #49(w1000) -> ()
        n566 = feedback #50(TRUE) -> (w1021:bool)
        n567 = case shown="2" "Operating Mode 2" {
          tunnel: [TRUE FALSE w1049] -> w1010
          tunnel: w1021 -> [_ _ w1046]
          frame 0, Default {
          }
          frame 1 {
          }
          frame 2 {
            n568 = Not(x=w1046) -> (.not. x?=w1048:bool)
            n569 = Select(t=w1048, s="Invert GI 2", f=w1046) -> (s? t:f=w1049:bool)
          }
        }
        n570 = And(x=w1010, y="Green FB On/Off") -> (x .and. y?=w1011:bool)
        n571 = case shown="True" w1011 {
          tunnel: "Current Out" -> [w1030 _]
          tunnel: [w1030 w1039] -> w1015
          frame False {
          }
          frame True {
            n572 = local read "Green FB Sum"() -> (w1035:i16)
            n573 = Bundle("P3"="P3", "I3"="I3", "D3"="D3") -> (w1031:cluster{"P3":i16, "I3":i16, "D3":i16})  [unwired: 1 in]
            n574 = call "Slower PID.vi"("process variable"=w1035, "reset?"="Green FB Reset", "setpoint"="Green FB Setpoint", "PID gains (x 2^8)"=w1031, "output range"=cluster{"output high":i16, "output low":i16} {"output high"=32767, "output low"=-32768} ("Green FB output range")) -> ("output"=w1042:i16)  [unwired: 10 out]
            n575 = To Long Integer(number=w1042) -> (32bit integer=w1036:i32)
            n576 = Add(x=w1036, y=32768) -> (x+y=w1038:i32)
            n577 = To Unsigned Word Integer(number=w1038) -> (unsigned 16bit integer=w1039:u16)
          }
        }
        n578 = Not(x=w1021) -> (.not. x?=w1018:bool)
        n579 = Select(t=w1009, s=w1018, f=w1008) -> (s? t:f=w1023:u16)
        n580 = Subtract(x=w1023, y=w992) -> (x-y=w1003:u16)
        n581 = Add(x=w1003, y=w1001) -> (x+y=w999:u16)
        n582 = feedback-in #50(w1018) -> ()
        n583 = Boolean To (0,1)(Boolean=w1010) -> (0, 1=w1017:i16)
        n584 = To Unsigned Word Integer(number=w1017) -> (unsigned 16bit integer=w1014:u16)
        n585 = Multiply(x=w1014, y=w1015) -> (x*y=w1016:u16)
      }
    }
  }
  n586 = while "532 nm green excitation laser intensity feedback measurement" {
    shift-right: [w1050] -> _
    shift-left: w2 -> [w1055]
    stop <- FALSE stop-if-true
    n587 = flat-sequence {
      tunnel: w1055 -> [w1057]
      tunnel: [w1058] -> w1053
      tunnel: [w1057] -> w1051
      tunnel: [w1062] -> w1054
      tunnel: w1053 -> [w1062]
      tunnel: [w1061] -> w1052
      tunnel: w1051 -> [w1061]
      tunnel: [w1074] -> w1050
      tunnel: w1054 -> [w1085]
      tunnel: w1052 -> [w1082]
      frame #0 {
        n588 = call "Loop Timer9"("Count(Ticks)"=w1057) -> ("Tick Count(Ticks)"=w1058:u16)
      }
      frame #1 {
        n589 = xnode "FPGA I/O Node"("Connector1/DIO35"=TRUE) -> ("Chassis2/Mod1/AI0"=→"Green FB Sum":i16)  [unwired: 2 in, 2 out]
      }
      frame #2 {
        n590 = feedback-in #51(w1085) -> ()
        n591 = feedback #51(w1085) -> (w1084:u16)
        n592 = Subtract(x=w1085, y=w1084) -> (x-y=w1083:u16)
        n593 = xnode "FPGA I/O Node"("Connector1/DIO35"=FALSE) -> ()  [unwired: 1 in, 1 out]
        n594 = Subtract(x=w1083, y=w1082) -> (x-y=w1064:u16)
        n595 = Subtract(x="Green FB Count", y=w1064) -> (x-y=w1078:u16)
        n596 = Number To Boolean Array(number=w1064) -> (Boolean array=w1065:bool[])
        n597 = Or Array Elements(Boolean array=w1065) -> (logical OR=w1063:bool)
        n598 = Boolean To (0,1)(Boolean="+ phase (Green FB)") -> (0, 1=w1076:i16)
        n599 = Boolean To (0,1)(Boolean=w1063) -> (0, 1=w1070:i16)
        n600 = Multiply(x=w1076, y="Phase count adjustment (Green FB)") -> (x*y=w1071:i16)
        n601 = Add(x=w1078, y=w1071) -> (x+y=w1074:u16)
        n602 = To Unsigned Byte Integer(number=w1070) -> (unsigned 8bit integer=w1067:u8)
        n603 = feedback #52(i16 0) -> (w1073:i16)
        n604 = Subtract(x=w1073, y=w1071) -> (x-y=w1072:i16)
        "Green FB Relative Phase" <- w1072
        n605 = feedback-in #52(w1072) -> ()
        n606 = feedback #53(u8 0) -> (w1068:u8)
        n607 = Add(x=w1067, y=w1068) -> (x+y=w1066:u8)
        "Green Late Counter" <- w1066
        n608 = feedback-in #53(w1066) -> ()
      }
    }
  }
  n609 = node-c288(w6) -> ()
  n610 = while "APD 3 Counter" {
    stop <- FALSE stop-if-true
    n611 = flat-sequence {
      frame #0 {
        n612 = xnode "FPGA I/O Method Node"("FPGA I/O In"=refnum<k21> "Connector0/DIO2" ("APD 2 DO"), "Timeout"=-1) -> ()  [unwired: 2 out]
      }
      frame #1 {
        n613 = local read "APD3 out state"() -> (w1089:bool)
        n614 = case shown="False" w1089 {
          frame False {
            n615 = local read "APD 3 Counts 0"() -> (w1091:u32)
            n616 = Increment(x=w1091) -> (x+1=→"APD 3 Counts 0":u32)
          }
          frame True {
            n617 = local read "APD 3 Counts 1"() -> (w1093:u32)
            n618 = Increment(x=w1093) -> (x+1=→"APD 3 Counts 1":u32)
          }
        }
      }
    }
  }
  n619 = while "APD 3 Gating" {
    shift-right: [w1097] -> _
    shift-left: w2 -> [w1102]
    shift-right: [w1096] -> _
    shift-left: w3 -> [w1094]
    stop <- FALSE stop-if-true
    n620 = flat-sequence {
      tunnel: w1102 -> [w1105]
      tunnel: [w1106] -> w1100
      tunnel: [w1105] -> w1098
      tunnel: [w1104] -> w1095
      tunnel: w1094 -> [w1104]
      tunnel: [w1109] -> w1101
      tunnel: w1100 -> [w1109]
      tunnel: [w1108] -> w1099
      tunnel: w1098 -> [w1108]
      tunnel: w1095 -> [w1107]
      tunnel: [w1126] -> w1097
      tunnel: w1101 -> [w1138]
      tunnel: w1099 -> [w1135]
      tunnel: [w1130] -> w1096
      frame #0 {
        n621 = call "Loop Timer15"("Count(Ticks)"=w1105) -> ("Tick Count(Ticks)"=w1106:u16)
      }
      frame #1 {
        # "Signal is then sent through \na transistor before APD"
        n622 = xnode "FPGA I/O Node"("Connector0/DIO9"=w1107) -> ()  [unwired: 1 in, 1 out]
      }
      frame #2 {
        n623 = local read "APD Gate OFF Count"() -> (w1111:u16)
        n624 = local read "APD Gate ON Count"() -> (w1112:u16)
        n625 = feedback #54(TRUE) -> (w1132:bool)
        n626 = feedback-in #55(w1138) -> ()
        n627 = feedback #55(w1138) -> (w1137:u16)
        n628 = Not(x=w1132) -> (.not. x?=w1129:bool)
        n629 = feedback-in #54(w1129) -> ()
        n630 = Subtract(x=w1138, y=w1137) -> (x-y=w1136:u16)
        n631 = Select(t=w1112, s=w1129, f=w1111) -> (s? t:f=w1134:u16)
        n632 = Subtract(x=w1136, y=w1135) -> (x-y=w1114:u16)
        n633 = Subtract(x=w1134, y=w1114) -> (x-y=w1125:u16)
        n634 = Number To Boolean Array(number=w1114) -> (Boolean array=w1115:bool[])
        n635 = Or Array Elements(Boolean array=w1115) -> (logical OR=w1113:bool)
        n636 = Boolean To (0,1)(Boolean=w1113) -> (0, 1=w1120:i16)
        n637 = Boolean To (0,1)(Boolean="+ phase (APD 3 Gate)") -> (0, 1=w1123:i16)
        n638 = To Unsigned Byte Integer(number=w1120) -> (unsigned 8bit integer=w1117:u8)
        n639 = Multiply(x=w1123, y="Phase count adjustment (APD 3 Gate)") -> (x*y=w1121:i16)
        n640 = feedback #56(u8 0) -> (w1118:u8)
        n641 = Add(x=w1117, y=w1118) -> (x+y=w1116:u8)
        "APD 3 Gate Late Counter" <- w1116
        n642 = feedback-in #56(w1116) -> ()
        n643 = Add(x=w1125, y=w1121) -> (x+y=w1126:u16)
        n644 = feedback #57(i16 0) -> (w1128:i16)
        n645 = Subtract(x=w1128, y=w1121) -> (x-y=w1127:i16)
        "APD 3 Gate Relative Phase" <- w1127
        n646 = feedback-in #57(w1127) -> ()
        n647 = local read "APD Gate Operating Mode"() -> (w1110:u8)
        n648 = case shown="2" w1110 {
          tunnel: [TRUE FALSE w1144] -> w1130
          tunnel: w1132 -> [_ _ w1142]
          frame 0, Default {
          }
          frame 1 {
          }
          frame 2 {
            n649 = local read "Invert APD Gate"() -> (w1141:bool)
            n650 = Not(x=w1142) -> (.not. x?=w1143:bool)
            n651 = Select(t=w1143, s=w1141, f=w1142) -> (s? t:f=w1144:bool)
          }
        }
      }
    }
  }
  n652 = while "Red fluorescent laser interlacing (Current to IA 633 nm AOM ME amp)." {
    shift-right: [w1150] -> _
    shift-left: w2 -> [w1153]
    shift-right: [w1147] -> _
    shift-left: w2 -> [w1145]
    stop <- FALSE stop-if-true
    n653 = flat-sequence {
      tunnel: w1153 -> [w1156]
      tunnel: [w1157] -> w1152
      tunnel: [w1156] -> w1151
      tunnel: [w1155] -> w1146
      tunnel: w1145 -> [w1155]
      tunnel: [w1160] -> w1149
      tunnel: w1152 -> [w1160]
      tunnel: [w1159] -> w1148
      tunnel: w1151 -> [w1159]
      tunnel: w1146 -> [w1158]
      tunnel: [w1169] -> w1150
      tunnel: [w1186] -> w1147
      tunnel: w1149 -> [w1199]
      tunnel: w1148 -> [w1196]
      frame #0 {
        n654 = call "Loop Timer2"("Count(Ticks)"=w1156) -> ("Tick Count(Ticks)"=w1157:u16)
      }
      frame #1 {
        n655 = xnode "FPGA I/O Node"("Chassis2/Mod4/AO1"=w1158) -> ()  [unwired: 1 in, 1 out]
      }
      frame #2 {
        n656 = Subtract(x="Red interlace OFF count 2", y="Red int current ON count adj") -> (x-y=w1178:u16)
        n657 = feedback-in #58(w1199) -> ()
        n658 = feedback #58(w1199) -> (w1198:u16)
        n659 = Add(x="Red int current ON count adj", y="Red interlace ON count 2") -> (x+y=w1179:u16)
        n660 = Subtract(x=w1199, y=w1198) -> (x-y=w1197:u16)
        n661 = Subtract(x=w1197, y=w1196) -> (x-y=w1162:u16)
        n662 = Number To Boolean Array(number=w1162) -> (Boolean array=w1163:bool[])
        n663 = Boolean To (0,1)(Boolean="+ phase (RI) 2") -> (0, 1=w1175:i16)
        n664 = Or Array Elements(Boolean array=w1163) -> (logical OR=w1161:bool)
        n665 = Boolean To (0,1)(Boolean=w1161) -> (0, 1=w1168:i16)
        n666 = Multiply(x=w1175, y="Phase count adjustment (RI) 2") -> (x*y=w1171:i16)
        n667 = To Unsigned Byte Integer(number=w1168) -> (unsigned 8bit integer=w1164:u8)
        n668 = feedback #59(u8 0) -> (w1166:u8)
        n669 = Add(x=w1164, y=w1166) -> (x+y=w1165:u8)
        "RI Late Counter 2" <- w1165
        n670 = feedback-in #59(w1165) -> ()
        n671 = feedback #60(i16 0) -> (w1172:i16)
        n672 = Subtract(x=w1172, y=w1171) -> (x-y=w1170:i16)
        "RI Relative phase 2" <- w1170
        n673 = feedback-in #60(w1170) -> ()
        n674 = feedback #61(TRUE) -> (w1191:bool)
        n675 = case shown="2" "RI Operating Mode 2" {
          tunnel: [TRUE FALSE w1219] -> w1180
          tunnel: w1191 -> [_ _ w1216]
          frame 0, Default {
          }
          frame 1 {
          }
          frame 2 {
            n676 = Not(x=w1216) -> (.not. x?=w1218:bool)
            n677 = Select(t=w1218, s="Invert RI 2", f=w1216) -> (s? t:f=w1219:bool)
          }
        }
        n678 = And(x=w1180, y="Red FB On/Off") -> (x .and. y?=w1181:bool)
        n679 = case shown="True" w1181 {
          tunnel: "RI Current Out" -> [w1200 _]
          tunnel: [w1200 w1209] -> w1185
          frame False {
          }
          frame True {
            n680 = local read "Red FB Intensity"() -> (w1205:i16)
            n681 = Bundle("P4"="P4", "I4"="I4", "D4"="D4") -> (w1201:cluster{"P4":i16, "I4":i16, "D4":i16})  [unwired: 1 in]
            n682 = call "Slower PID.vi"("process variable"=w1205, "reset?"="Red FB Reset", "setpoint"="Red FB Setpoint", "PID gains (x 2^8)"=w1201, "output range"=cluster{"output high":i16, "output low":i16} {"output high"=32767, "output low"=-32768} ("Green FB output range")) -> ("output"=w1212:i16)  [unwired: 10 out]
            n683 = To Long Integer(number=w1212) -> (32bit integer=w1206:i32)
            n684 = Add(x=w1206, y=32768) -> (x+y=w1208:i32)
            n685 = To Unsigned Word Integer(number=w1208) -> (unsigned 16bit integer=w1209:u16)
          }
        }
        n686 = Not(x=w1191) -> (.not. x?=w1188:bool)
        n687 = Select(t=w1179, s=w1188, f=w1178) -> (s? t:f=w1193:u16)
        n688 = Subtract(x=w1193, y=w1162) -> (x-y=w1173:u16)
        n689 = Add(x=w1173, y=w1171) -> (x+y=w1169:u16)
        n690 = feedback-in #61(w1188) -> ()
        n691 = Boolean To (0,1)(Boolean=w1180) -> (0, 1=w1187:i16)
        n692 = To Unsigned Word Integer(number=w1187) -> (unsigned 16bit integer=w1184:u16)
        n693 = Multiply(x=w1184, y=w1185) -> (x*y=w1186:u16)
      }
    }
  }
  n694 = while "633 nm red excitation laser intensity feedback measurement" {
    shift-right: [w1220] -> _
    shift-left: w2 -> [w1225]
    stop <- FALSE stop-if-true
    n695 = flat-sequence {
      tunnel: w1225 -> [w1227]
      tunnel: [w1228] -> w1223
      tunnel: [w1227] -> w1221
      tunnel: [w1232] -> w1224
      tunnel: w1223 -> [w1232]
      tunnel: [w1231] -> w1222
      tunnel: w1221 -> [w1231]
      tunnel: [w1244] -> w1220
      tunnel: w1224 -> [w1255]
      tunnel: w1222 -> [w1252]
      frame #0 {
        n696 = call "Loop Timer12"("Count(Ticks)"=w1227) -> ("Tick Count(Ticks)"=w1228:u16)
      }
      frame #1 {
        n697 = xnode "FPGA I/O Node"("Connector1/DIO29"=TRUE ("Connector1/DIO35")) -> ("Chassis2/Mod1/AI1"=→"Red FB Intensity":i16)  [unwired: 2 in, 2 out]
      }
      frame #2 {
        n698 = feedback-in #62(w1255) -> ()
        n699 = feedback #62(w1255) -> (w1254:u16)
        n700 = Subtract(x=w1255, y=w1254) -> (x-y=w1253:u16)
        n701 = xnode "FPGA I/O Node"("Connector1/DIO29"=FALSE ("Connector1/DIO35")) -> ()  [unwired: 1 in, 1 out]
        n702 = Subtract(x=w1253, y=w1252) -> (x-y=w1234:u16)
        n703 = Subtract(x="Red FB Count", y=w1234) -> (x-y=w1248:u16)
        n704 = Number To Boolean Array(number=w1234) -> (Boolean array=w1235:bool[])
        n705 = Or Array Elements(Boolean array=w1235) -> (logical OR=w1233:bool)
        n706 = Boolean To (0,1)(Boolean="+ phase (Red FB)") -> (0, 1=w1246:i16)
        n707 = Boolean To (0,1)(Boolean=w1233) -> (0, 1=w1240:i16)
        n708 = Multiply(x=w1246, y="Phase count adjustment (Red FB)") -> (x*y=w1241:i16)
        n709 = Add(x=w1248, y=w1241) -> (x+y=w1244:u16)
        n710 = To Unsigned Byte Integer(number=w1240) -> (unsigned 8bit integer=w1237:u8)
        n711 = feedback #63(i16 0) -> (w1243:i16)
        n712 = Subtract(x=w1243, y=w1241) -> (x-y=w1242:i16)
        "Red FB Relative Phase" <- w1242
        n713 = feedback-in #63(w1242) -> ()
        n714 = feedback #64(u8 0) -> (w1238:u8)
        n715 = Add(x=w1237, y=w1238) -> (x+y=w1236:u8)
        "Red Late Counter" <- w1236
        n716 = feedback-in #64(w1236) -> ()
      }
    }
  }
  n717 = while "633 nm red  fluorescent laser interlacing (DO to IA 633 nm AOM ME amp)." {
    shift-right: [w1259] -> _
    shift-left: w2 -> [w1264]
    shift-right: [w1258] -> _
    shift-left: _ -> [w1256]
    stop <- FALSE stop-if-true
    n718 = flat-sequence {
      tunnel: w1264 -> [w1267]
      tunnel: [w1268] -> w1262
      tunnel: [w1267] -> w1260
      tunnel: [w1266] -> w1257
      tunnel: w1256 -> [w1266]
      tunnel: [w1271] -> w1263
      tunnel: w1262 -> [w1271]
      tunnel: [w1270] -> w1261
      tunnel: w1260 -> [w1270]
      tunnel: w1257 -> [w1269]
      tunnel: [w1280] -> w1259
      tunnel: w1263 -> [w1300]
      tunnel: w1261 -> [w1297]
      tunnel: [w1289] -> w1258
      frame #0 {
        n719 = call "Loop Timer11"("Count(Ticks)"=w1267) -> ("Tick Count(Ticks)"=w1268:u16)
      }
      frame #1 {
        # "Then to PRL 440 amp"
        n720 = xnode "FPGA I/O Node"("Connector1/DIO32"=w1269) -> ()  [unwired: 1 in, 1 out]
      }
      frame #2 {
        n721 = feedback-in #65(w1300) -> ()
        n722 = feedback #65(w1300) -> (w1299:u16)
        n723 = Subtract(x=w1300, y=w1299) -> (x-y=w1298:u16)
        n724 = Subtract(x=w1298, y=w1297) -> (x-y=w1273:u16)
        n725 = Number To Boolean Array(number=w1273) -> (Boolean array=w1274:bool[])
        n726 = Or Array Elements(Boolean array=w1274) -> (logical OR=w1272:bool)
        n727 = Boolean To (0,1)(Boolean="+ phase (RI)") -> (0, 1=w1285:i16)
        n728 = Multiply(x=w1285, y="Phase count adjustment (RI)") -> (x*y=w1282:i16)
        n729 = Boolean To (0,1)(Boolean=w1272) -> (0, 1=w1279:i16)
        n730 = To Unsigned Byte Integer(number=w1279) -> (unsigned 8bit integer=w1276:u8)
        n731 = feedback #66(i16 0) -> (w1283:i16)
        n732 = feedback #67(u8 0) -> (w1277:u8)
        n733 = Add(x=w1276, y=w1277) -> (x+y=w1275:u8)
        "RI Late Counter" <- w1275
        n734 = feedback-in #67(w1275) -> ()
        n735 = Subtract(x=w1283, y=w1282) -> (x-y=w1281:i16)
        "RI Relative phase" <- w1281
        n736 = feedback-in #66(w1281) -> ()
        n737 = feedback #68(TRUE) -> (w1292:bool)
        n738 = case shown="2" "Red Laser Operating Mode" {
          tunnel: [TRUE FALSE w1306] -> w1289
          tunnel: w1292 -> [_ _ w1303]
          frame 0, Default {
          }
          frame 1 {
          }
          frame 2 {
            n739 = Not(x=w1303) -> (.not. x?=w1305:bool)
            n740 = Select(t=w1305, s="Invert RI", f=w1303) -> (s? t:f=w1306:bool)
          }
        }
        n741 = Not(x=w1292) -> (.not. x?=w1288:bool)
        n742 = Select(t="Red interlace ON count", s=w1288, f="Red interlace OFF count") -> (s? t:f=w1294:u16)
        n743 = Subtract(x=w1294, y=w1273) -> (x-y=w1286:u16)
        n744 = Add(x=w1286, y=w1282) -> (x+y=w1280:u16)
        n745 = feedback-in #68(w1288) -> ()
      }
    }
  }
  n746 = while "473 nm blue excitation laser intensity feedback measurement" {
    shift-right: [w1307] -> _
    shift-left: w2 -> [w1312]
    stop <- FALSE stop-if-true
    n747 = flat-sequence {
      tunnel: w1312 -> [w1314]
      tunnel: [w1315] -> w1310
      tunnel: [w1314] -> w1308
      tunnel: [w1319] -> w1311
      tunnel: w1310 -> [w1319]
      tunnel: [w1318] -> w1309
      tunnel: w1308 -> [w1318]
      tunnel: [w1332] -> w1307
      tunnel: w1311 -> [w1342]
      tunnel: w1309 -> [w1339]
      frame #0 {
        n748 = call "Loop Timer16"("Count(Ticks)"=w1314) -> ("Tick Count(Ticks)"=w1315:u16)
      }
      frame #1 {
        # "Removed analog in."
        n749 = xnode "FPGA I/O Node"("Connector1/DIO34"=TRUE ("Connector0/DIO11")) -> ()  [unwired: 1 in, 1 out]
        "Blue Intensity" <- i16 0 ("Blue Intensity")
      }
      frame #2 {
        n750 = feedback-in #69(w1342) -> ()
        n751 = feedback #69(w1342) -> (w1341:u16)
        n752 = Subtract(x=w1342, y=w1341) -> (x-y=w1340:u16)
        n753 = xnode "FPGA I/O Node"("Connector1/DIO34"=FALSE ("Connector0/DIO11")) -> ()  [unwired: 1 in, 1 out]
        n754 = Subtract(x=w1340, y=w1339) -> (x-y=w1322:u16)
        n755 = Subtract(x="Blue Int Count", y=w1322) -> (x-y=w1336:u16)
        n756 = Number To Boolean Array(number=w1322) -> (Boolean array=w1323:bool[])
        n757 = Or Array Elements(Boolean array=w1323) -> (logical OR=w1321:bool)
        n758 = Boolean To (0,1)(Boolean=w1321) -> (0, 1=w1328:i16)
        n759 = Boolean To (0,1)(Boolean="+ phase (Blue Int)") -> (0, 1=w1334:i16)
        n760 = To Unsigned Byte Integer(number=w1328) -> (unsigned 8bit integer=w1325:u8)
        n761 = Multiply(x=w1334, y="Phase count adjustment (Blue Int)") -> (x*y=w1329:i16)
        n762 = feedback #70(u8 0) -> (w1326:u8)
        n763 = Add(x=w1325, y=w1326) -> (x+y=w1324:u8)
        "Blue Int Late Counter" <- w1324
        n764 = feedback-in #70(w1324) -> ()
        n765 = Add(x=w1336, y=w1329) -> (x+y=w1332:u16)
        n766 = feedback #71(i16 0) -> (w1331:i16)
        n767 = Subtract(x=w1331, y=w1329) -> (x-y=w1330:i16)
        "Blue Int Relative Phase" <- w1330
        n768 = feedback-in #71(w1330) -> ()
      }
    }
  }
  n769 = while "473 nm blue  fluorescent laser interlacing (DO to blue laser digital control input)." {
    shift-right: [w1346] -> _
    shift-left: w2 -> [w1351]
    shift-right: [w1345] -> _
    shift-left: _ -> [w1343]
    stop <- FALSE stop-if-true
    n770 = flat-sequence {
      tunnel: w1351 -> [w1354]
      tunnel: [w1355] -> w1349
      tunnel: [w1354] -> w1347
      tunnel: [w1353] -> w1344
      tunnel: w1343 -> [w1353]
      tunnel: [w1358] -> w1350
      tunnel: w1349 -> [w1358]
      tunnel: [w1357] -> w1348
      tunnel: w1347 -> [w1357]
      tunnel: w1344 -> [w1356]
      tunnel: [w1367] -> w1346
      tunnel: w1350 -> [w1387]
      tunnel: w1348 -> [w1384]
      tunnel: [w1376] -> w1345
      frame #0 {
        n771 = call "Loop Timer14"("Count(Ticks)"=w1354) -> ("Tick Count(Ticks)"=w1355:u16)
      }
      frame #1 {
        n772 = xnode "FPGA I/O Node"("Connector1/DIO28"=w1356) -> ()  [unwired: 1 in, 1 out]
      }
      frame #2 {
        n773 = feedback-in #72(w1387) -> ()
        n774 = feedback #72(w1387) -> (w1386:u16)
        n775 = Subtract(x=w1387, y=w1386) -> (x-y=w1385:u16)
        n776 = Subtract(x=w1385, y=w1384) -> (x-y=w1360:u16)
        n777 = Number To Boolean Array(number=w1360) -> (Boolean array=w1361:bool[])
        n778 = Or Array Elements(Boolean array=w1361) -> (logical OR=w1359:bool)
        n779 = Boolean To (0,1)(Boolean="+ phase (BI D)") -> (0, 1=w1372:i16)
        n780 = Multiply(x=w1372, y="Phase count adjustment (BI D)") -> (x*y=w1369:i16)
        n781 = Boolean To (0,1)(Boolean=w1359) -> (0, 1=w1366:i16)
        n782 = To Unsigned Byte Integer(number=w1366) -> (unsigned 8bit integer=w1363:u8)
        n783 = feedback #73(i16 0) -> (w1370:i16)
        n784 = feedback #74(u8 0) -> (w1364:u8)
        n785 = Add(x=w1363, y=w1364) -> (x+y=w1362:u8)
        "Blue Late Counter (D)" <- w1362
        n786 = feedback-in #74(w1362) -> ()
        n787 = Subtract(x=w1370, y=w1369) -> (x-y=w1368:i16)
        "BI Relative phase (D)" <- w1368
        n788 = feedback-in #73(w1368) -> ()
        n789 = feedback #75(TRUE) -> (w1379:bool)
        n790 = case shown="2" "Blue Laser Operating Mode (D)" {
          tunnel: [TRUE FALSE w1393] -> w1376
          tunnel: w1379 -> [_ _ w1390]
          frame 0, Default {
          }
          frame 1 {
          }
          frame 2 {
            n791 = Not(x=w1390) -> (.not. x?=w1392:bool)
            n792 = Select(t=w1392, s="Invert BI (D)", f=w1390) -> (s? t:f=w1393:bool)
          }
        }
        n793 = Not(x=w1379) -> (.not. x?=w1375:bool)
        n794 = Select(t="Blue interlace ON count (D)", s=w1375, f="Blue interlace OFF count (D)") -> (s? t:f=w1381:u16)
        n795 = Subtract(x=w1381, y=w1360) -> (x-y=w1373:u16)
        n796 = Add(x=w1373, y=w1369) -> (x+y=w1367:u16)
        n797 = feedback-in #75(w1375) -> ()
      }
    }
  }
  n798 = while "Blue fluorescent laser interlacing (AO control direct to laser)." {
    shift-right: [w1399] -> _
    shift-left: w2 -> [w1402]
    shift-right: [w1396] -> _
    shift-left: i16 0 -> [w1394]
    stop <- FALSE stop-if-true
    n799 = flat-sequence {
      tunnel: w1402 -> [w1405]
      tunnel: [w1406] -> w1401
      tunnel: [w1405] -> w1400
      tunnel: [w1404] -> w1395
      tunnel: w1394 -> [w1404]
      tunnel: [w1409] -> w1398
      tunnel: w1401 -> [w1409]
      tunnel: [w1408] -> w1397
      tunnel: w1400 -> [w1408]
      tunnel: w1395 -> [w1407]
      tunnel: [w1419] -> w1399
      tunnel: [w1435] -> w1396
      tunnel: w1398 -> [w1447]
      tunnel: w1397 -> [w1444]
      frame #0 {
        n800 = call "Loop Timer13"("Count(Ticks)"=w1405) -> ("Tick Count(Ticks)"=w1406:u16)
      }
      frame #1 {
        n801 = xnode "FPGA I/O Node"("Connector0/AO3"=w1407) -> ()  [unwired: 1 in, 1 out]
      }
      frame #2 {
        n802 = Subtract(x="Blue OFF count (AO)", y="Blue current ON count adj (AO)") -> (x-y=w1428:u16)
        n803 = feedback-in #76(w1447) -> ()
        n804 = feedback #76(w1447) -> (w1446:u16)
        n805 = Add(x="Blue current ON count adj (AO)", y="Blue ON count (AO)") -> (x+y=w1429:u16)
        n806 = Subtract(x=w1447, y=w1446) -> (x-y=w1445:u16)
        n807 = Subtract(x=w1445, y=w1444) -> (x-y=w1412:u16)
        n808 = Number To Boolean Array(number=w1412) -> (Boolean array=w1413:bool[])
        n809 = Boolean To (0,1)(Boolean="+ phase (BI AO)") -> (0, 1=w1425:i16)
        n810 = Or Array Elements(Boolean array=w1413) -> (logical OR=w1411:bool)
        n811 = Boolean To (0,1)(Boolean=w1411) -> (0, 1=w1418:i16)
        n812 = Multiply(x=w1425, y="Phase count adjustment (BI AO)") -> (x*y=w1421:i16)
        n813 = To Unsigned Byte Integer(number=w1418) -> (unsigned 8bit integer=w1414:u8)
        n814 = feedback #77(u8 0) -> (w1416:u8)
        n815 = Add(x=w1414, y=w1416) -> (x+y=w1415:u8)
        "BI Late Counter (AO)" <- w1415
        n816 = feedback-in #77(w1415) -> ()
        n817 = feedback #78(i16 0) -> (w1422:i16)
        n818 = Subtract(x=w1422, y=w1421) -> (x-y=w1420:i16)
        "BI Relative phase (AO)" <- w1420
        n819 = feedback-in #78(w1420) -> ()
        n820 = feedback #79(TRUE) -> (w1439:bool)
        n821 = case shown="2" "BI Operating Mode (AO)" {
          tunnel: [TRUE FALSE w1463] -> w1430
          tunnel: w1439 -> [_ _ w1460]
          frame 0, Default {
          }
          frame 1 {
          }
          frame 2 {
            n822 = Not(x=w1460) -> (.not. x?=w1462:bool)
            n823 = Select(t=w1462, s="Invert BI (AO)", f=w1460) -> (s? t:f=w1463:bool)
          }
        }
        n824 = And(x=w1430, y="Blue FB On/Off") -> (x .and. y?=w1431:bool)
        n825 = case shown="True" w1431 {
          tunnel: "BI Current Out" -> [w1448 _]
          tunnel: [w1448 w1450] -> w1434
          frame False {
          }
          frame True {
            n826 = local read "Blue Intensity"() -> (w1449:i16)
            n827 = Bundle("P5"="P5", "I5"="I5", "D5"="D5") -> (w1451:cluster{"P5":i16, "I5":i16, "D5":i16})  [unwired: 1 in]
            n828 = call "Slower PID.vi"("process variable"=w1449, "reset?"="Blue FB Reset", "setpoint"="Blue FB Setpoint", "PID gains (x 2^8)"=w1451, "output range"=cluster{"output high":i16, "output low":i16} {"output high"=32767, "output low"=0} ("Green FB output range")) -> ("output"=w1450:i16)  [unwired: 10 out]
          }
        }
        n829 = Not(x=w1439) -> (.not. x?=w1436:bool)
        n830 = Select(t=w1429, s=w1436, f=w1428) -> (s? t:f=w1441:u16)
        n831 = Subtract(x=w1441, y=w1412) -> (x-y=w1423:u16)
        n832 = Add(x=w1423, y=w1421) -> (x+y=w1419:u16)
        n833 = feedback-in #79(w1436) -> ()
        n834 = Boolean To (0,1)(Boolean=w1430) -> (0, 1=w1410:i16)
        n835 = Multiply(x=w1410, y=w1434) -> (x*y=w1435:i16)
      }
    }
  }
